vi "FormatDades.vi"(8 "Captador":refnum<vi>, 9 "Escala":u8, 10 "ValorIn":dbl, 11 "Unidades":refnum<vi>) -> (0 "NDecimals":u8, 2 "ValorOut":dbl)   [LabVIEW 2017]
panel:
  out "Value":u16
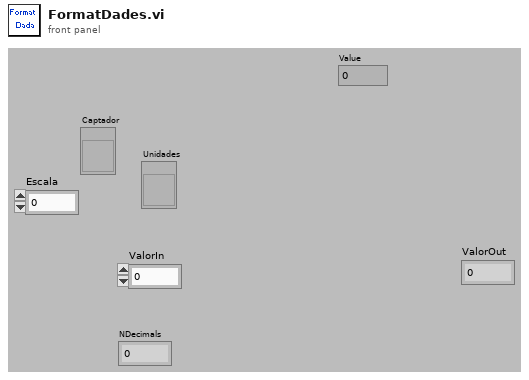
[diagram p1: front panel]
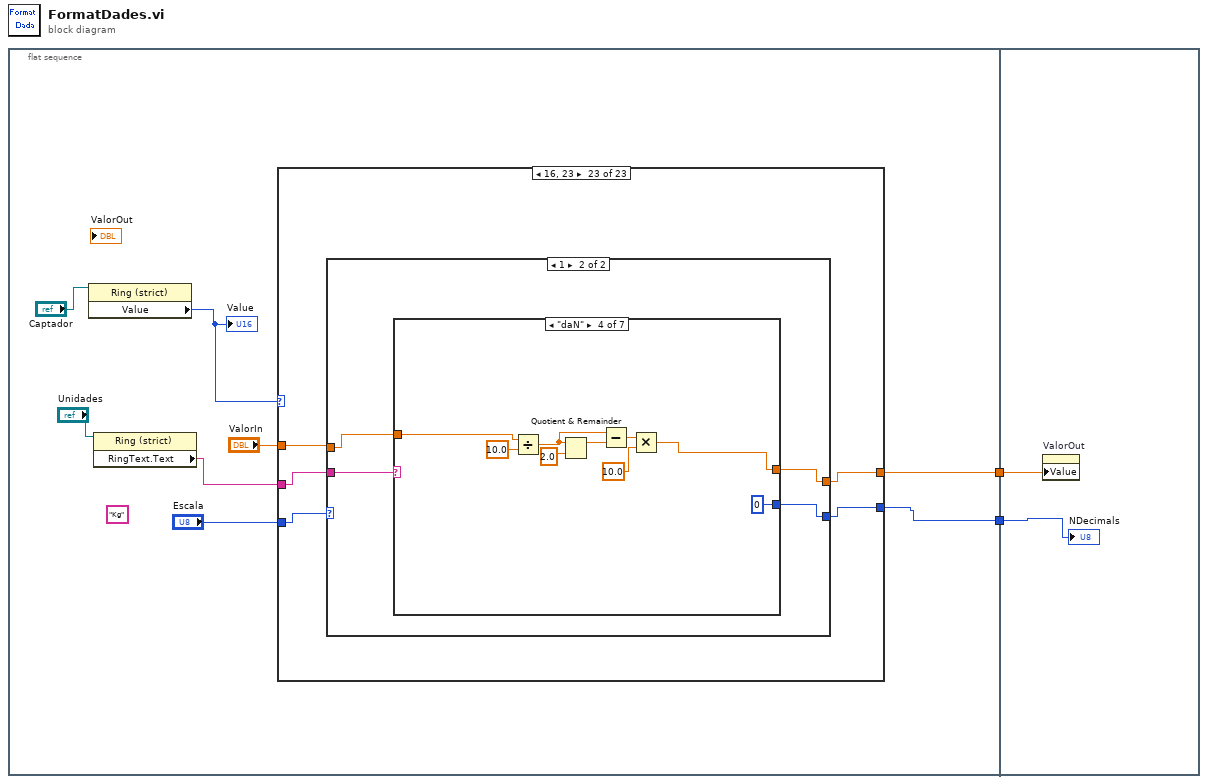
[diagram p0: block diagram]
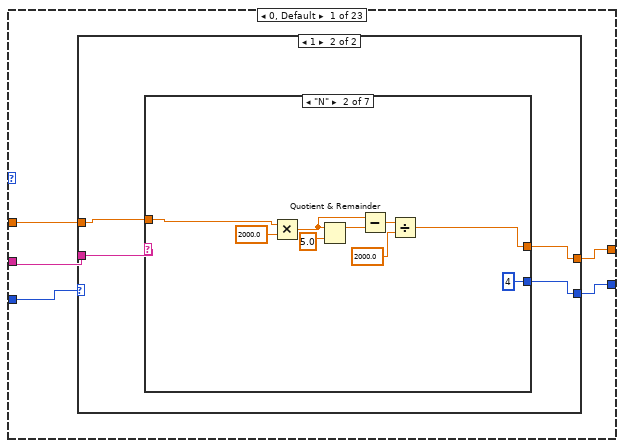
[diagram p2: hidden frame]
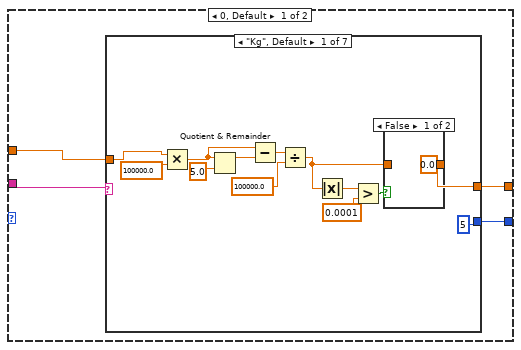
[diagram p3: hidden frame]
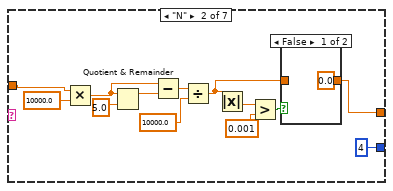
[diagram p5: hidden frame]
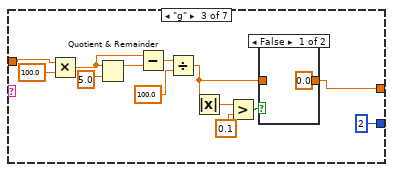
[diagram p7: hidden frame]
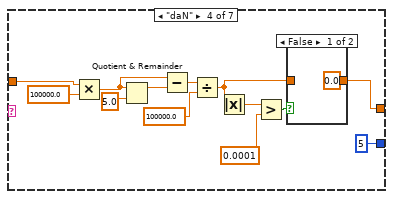
[diagram p9: hidden frame]
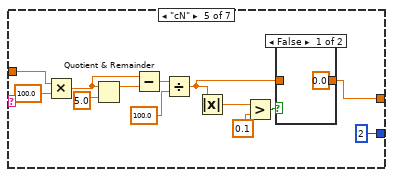
[diagram p11: hidden frame]
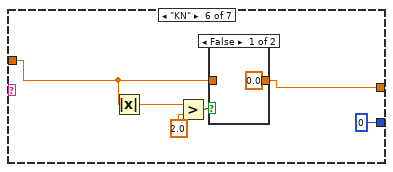
[diagram p13: hidden frame]
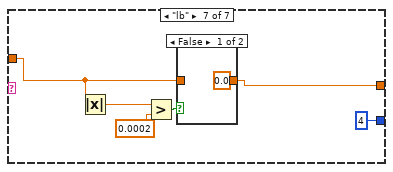
[diagram p15: hidden frame]
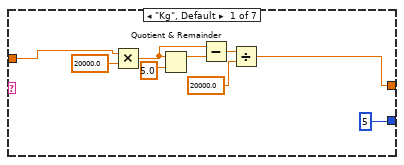
[diagram p17: hidden frame]
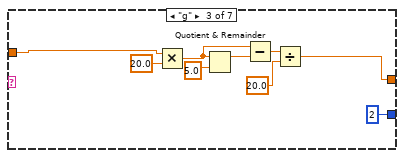
[diagram p18: hidden frame]
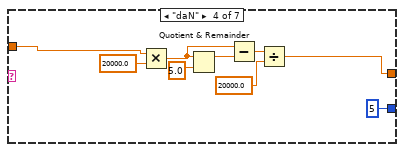
[diagram p19: hidden frame]
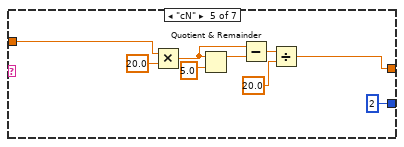
[diagram p20: hidden frame]
diagram:
  n1 = flat-sequence {
    tunnel: [w8] -> w2
    tunnel: [w3] -> w1
    tunnel: w2 -> [w3014]
    tunnel: w1 -> [w3013]
    frame #0 {
      (unwired) "Kg" ("RingText.Text")
      n2 = property class="Ring (strict)"(reference="Captador") -> ("Value"=w4:u16)  [unwired: 1 in, 2 out]
      "Value" <- w4
      n3 = property class="Ring (strict)"(reference="Unidades") -> ("RingText.Text"=w5:string)  [unwired: 1 in, 2 out]
      n4 = case shown="16, 23" w4 {
        tunnel: w5 -> [w15 w174 w293 w419 w573 w692 w819 w959 w1113 w1218 w1345 w1472 w1605 w1732 w1897 w2074 w2215 w2321 w2444 w2572 w2675 w2790 w2898]
        tunnel: [w14 w172 w291 w417 w571 w690 w816 w957 w1111 w1216 w1343 w1470 w1603 w1730 w1895 w2071 w2213 w2318 w2442 w2570 w2673 w2787 w2896] -> w8
        tunnel: "ValorIn" -> [w13 w175 w294 w420 w574 w693 w820 w960 w1114 w1219 w1346 w1473 w1606 w1733 w1898 w2075 w2216 w2322 w2445 w2573 w2676 w2791 w2899]
        tunnel: "Escala" -> [w12 w173 w292 w418 w572 w691 w818 w958 w1112 w1217 w1344 w1471 w1604 w1731 w1896 w2073 w2214 w2320 w2443 w2571 w2674 w2789 w2897]
        tunnel: [w11 w171 w290 w416 w570 w689 w817 w956 w1110 w1215 w1342 w1469 w1602 w1729 w1894 w2072 w2212 w2319 w2441 w2569 w2672 w2788 w2895] -> w3
        frame 0, Default {
          n5 = case shown="1" w12 {
            tunnel: w15 -> [w19 w113]
            tunnel: [w18 w112] -> w14
            tunnel: w13 -> [w17 w114]
            tunnel: [w16 w111] -> w11
            frame 0, Default {
              n6 = case shown="\"Kg\", Default" w19 {
                tunnel: [w21 w36 w52 w66 w81 w97 w105] -> w18
                tunnel: w17 -> [w25 w40 w55 w70 w86 w96 w104]
                tunnel: [5 4 2 5 2 0 4] -> w16
                frame "Kg", Default {
                  n7 = Multiply(x=w25, y=100000.0) -> (x*y=w28:dbl)
                  n8 = Quotient & Remainder(x=w28, y=5.0) -> (x-y*floor(x/y)=w29:dbl)  [unwired: 1 out]
                  n9 = Subtract(x=w28, y=w29) -> (x-y=w27:dbl)
                  n10 = Divide(x=w27, y=100000.0) -> (x/y=w22:dbl)
                  n11 = Absolute Value(x=w22) -> (abs(x)=w20:dbl)
                  n12 = Greater?(x=w20, y=0.0001) -> (0:w23:bool)
                  n13 = case shown="False" w23 {
                    tunnel: w22 -> [_ w34]
                    tunnel: [0.0 w34] -> w21
                    frame False {
                    }
                    frame True {
                    }
                  }
                }
                frame "N" {
                  n14 = Multiply(x=w40, y=10000.0) -> (x*y=w43:dbl)
                  n15 = Quotient & Remainder(x=w43, y=5.0) -> (x-y*floor(x/y)=w44:dbl)  [unwired: 1 out]
                  n16 = Subtract(x=w43, y=w44) -> (x-y=w42:dbl)
                  n17 = Divide(x=w42, y=10000.0) -> (x/y=w37:dbl)
                  n18 = Absolute Value(x=w37) -> (abs(x)=w35:dbl)
                  n19 = Greater?(x=w35, y=0.001) -> (0:w38:bool)
                  n20 = case shown="False" w38 {
                    tunnel: w37 -> [_ w49]
                    tunnel: [0.0 w49] -> w36
                    frame False {
                    }
                    frame True {
                    }
                  }
                }
                frame "g" {
                  n21 = Multiply(x=w55, y=100.0) -> (x*y=w58:dbl)
                  n22 = Quotient & Remainder(x=w58, y=5.0) -> (x-y*floor(x/y)=w59:dbl)  [unwired: 1 out]
                  n23 = Subtract(x=w58, y=w59) -> (x-y=w57:dbl)
                  n24 = Divide(x=w57, y=100.0) -> (x/y=w51:dbl)
                  n25 = Absolute Value(x=w51) -> (abs(x)=w50:dbl)
                  n26 = Greater?(x=w50, y=0.1) -> (0:w53:bool)
                  n27 = case shown="False" w53 {
                    tunnel: w51 -> [_ w64]
                    tunnel: [0.0 w64] -> w52
                    frame False {
                    }
                    frame True {
                    }
                  }
                }
                frame "daN" {
                  n28 = Multiply(x=w70, y=100000.0) -> (x*y=w73:dbl)
                  n29 = Quotient & Remainder(x=w73, y=5.0) -> (x-y*floor(x/y)=w74:dbl)  [unwired: 1 out]
                  n30 = Subtract(x=w73, y=w74) -> (x-y=w72:dbl)
                  n31 = Divide(x=w72, y=100000.0) -> (x/y=w67:dbl)
                  n32 = Absolute Value(x=w67) -> (abs(x)=w65:dbl)
                  n33 = Greater?(x=w65, y=0.0001) -> (0:w68:bool)
                  n34 = case shown="False" w68 {
                    tunnel: w67 -> [_ w79]
                    tunnel: [0.0 w79] -> w66
                    frame False {
                    }
                    frame True {
                    }
                  }
                }
                frame "cN" {
                  n35 = Multiply(x=w86, y=100.0) -> (x*y=w89:dbl)
                  n36 = Quotient & Remainder(x=w89, y=5.0) -> (x-y*floor(x/y)=w90:dbl)  [unwired: 1 out]
                  n37 = Subtract(x=w89, y=w90) -> (x-y=w88:dbl)
                  n38 = Divide(x=w88, y=100.0) -> (x/y=w82:dbl)
                  n39 = Absolute Value(x=w82) -> (abs(x)=w80:dbl)
                  n40 = Greater?(x=w80, y=0.1) -> (0:w83:bool)
                  n41 = case shown="False" w83 {
                    tunnel: w82 -> [_ w94]
                    tunnel: [0.0 w94] -> w81
                    frame False {
                    }
                    frame True {
                    }
                  }
                }
                frame "KN" {
                  n42 = Absolute Value(x=w96) -> (abs(x)=w95:dbl)
                  n43 = Greater?(x=w95, y=2.0) -> (0:w98:bool)
                  n44 = case shown="False" w98 {
                    tunnel: w96 -> [_ w102]
                    tunnel: [0.0 w102] -> w97
                    frame False {
                    }
                    frame True {
                    }
                  }
                }
                frame "lb" {
                  n45 = Absolute Value(x=w104) -> (abs(x)=w103:dbl)
                  n46 = Greater?(x=w103, y=0.0002) -> (0:w106:bool)
                  n47 = case shown="False" w106 {
                    tunnel: w104 -> [_ w110]
                    tunnel: [0.0 w110] -> w105
                    frame False {
                    }
                    frame True {
                    }
                  }
                }
              }
            }
            frame 1 {
              n48 = case shown="\"N\"" w113 {
                tunnel: [w115 w124 w133 w143 w153 w161 w162] -> w112
                tunnel: w114 -> [w116 w125 w134 w142 w152 w161 w163]
                tunnel: [5 4 2 5 2 0 4] -> w111
                frame "Kg", Default {
                  n49 = Multiply(x=w116, y=20000.0) -> (x*y=w119:dbl)
                  n50 = Quotient & Remainder(x=w119, y=5.0) -> (x-y*floor(x/y)=w120:dbl)  [unwired: 1 out]
                  n51 = Subtract(x=w119, y=w120) -> (x-y=w118:dbl)
                  n52 = Divide(x=w118, y=20000.0) -> (x/y=w115:dbl)
                }
                frame "N" {
                  n53 = Multiply(x=w125, y=2000.0) -> (x*y=w128:dbl)
                  n54 = Quotient & Remainder(x=w128, y=5.0) -> (x-y*floor(x/y)=w129:dbl)  [unwired: 1 out]
                  n55 = Subtract(x=w128, y=w129) -> (x-y=w127:dbl)
                  n56 = Divide(x=w127, y=2000.0) -> (x/y=w124:dbl)
                }
                frame "g" {
                  n57 = Multiply(x=w134, y=20.0) -> (x*y=w137:dbl)
                  n58 = Quotient & Remainder(x=w137, y=5.0) -> (x-y*floor(x/y)=w138:dbl)  [unwired: 1 out]
                  n59 = Subtract(x=w137, y=w138) -> (x-y=w136:dbl)
                  n60 = Divide(x=w136, y=20.0) -> (x/y=w133:dbl)
                }
                frame "daN" {
                  n61 = Multiply(x=w142, y=20000.0) -> (x*y=w146:dbl)
                  n62 = Quotient & Remainder(x=w146, y=5.0) -> (x-y*floor(x/y)=w147:dbl)  [unwired: 1 out]
                  n63 = Subtract(x=w146, y=w147) -> (x-y=w145:dbl)
                  n64 = Divide(x=w145, y=20000.0) -> (x/y=w143:dbl)
                }
                frame "cN" {
                  n65 = Multiply(x=w152, y=20.0) -> (x*y=w156:dbl)
                  n66 = Quotient & Remainder(x=w156, y=5.0) -> (x-y*floor(x/y)=w157:dbl)  [unwired: 1 out]
                  n67 = Subtract(x=w156, y=w157) -> (x-y=w155:dbl)
                  n68 = Divide(x=w155, y=20.0) -> (x/y=w153:dbl)
                }
                frame "KN" {
                }
                frame "lb" {
                  n69 = Multiply(x=w163, y=10000.0) -> (x*y=w166:dbl)
                  n70 = Quotient & Remainder(x=w166, y=5.0) -> (x-y*floor(x/y)=w167:dbl)  [unwired: 1 out]
                  n71 = Subtract(x=w166, y=w167) -> (x-y=w165:dbl)
                  n72 = Divide(x=w165, y=10000.0) -> (x/y=w162:dbl)
                }
              }
            }
          }
        }
        frame 1 {
          n73 = case shown="0, Default" w173 {
            tunnel: [w179 w240] -> w172
            tunnel: [w178 w239] -> w171
            tunnel: w175 -> [w177 w238]
            tunnel: w174 -> [w176 w237]
            frame 0, Default {
              n74 = case shown="\"Kg\", Default" w176 {
                tunnel: [w181 w189 w197 w205 w213 w220 w223] -> w179
                tunnel: [4 3 1 4 1 0 4] -> w178
                tunnel: w177 -> [w182 w190 w198 w206 w214 w220 w227]
                frame "Kg", Default {
                  n75 = Absolute Value(x=w182) -> (abs(x)=w180:dbl)
                  n76 = Greater?(x=w180, y=0.0002) -> (0:w183:bool)
                  n77 = case shown="False" w183 {
                    tunnel: w182 -> [_ w187]
                    tunnel: [0.0 w187] -> w181
                    frame False {
                    }
                    frame True {
                    }
                  }
                }
                frame "N" {
                  n78 = Absolute Value(x=w190) -> (abs(x)=w188:dbl)
                  n79 = Greater?(x=w188, y=0.002) -> (0:w191:bool)
                  n80 = case shown="False" w191 {
                    tunnel: w190 -> [_ w195]
                    tunnel: [0.0 w195] -> w189
                    frame False {
                    }
                    frame True {
                    }
                  }
                }
                frame "g" {
                  n81 = Absolute Value(x=w198) -> (abs(x)=w196:dbl)
                  n82 = Greater?(x=w196, y=2.0) -> (0:w199:bool)
                  n83 = case shown="False" w199 {
                    tunnel: w198 -> [_ w203]
                    tunnel: [0.0 w203] -> w197
                    frame False {
                    }
                    frame True {
                    }
                  }
                }
                frame "daN" {
                  n84 = Absolute Value(x=w206) -> (abs(x)=w204:dbl)
                  n85 = Greater?(x=w204, y=0.0002) -> (0:w207:bool)
                  n86 = case shown="False" w207 {
                    tunnel: w206 -> [_ w211]
                    tunnel: [0.0 w211] -> w205
                    frame False {
                    }
                    frame True {
                    }
                  }
                }
                frame "cN" {
                  n87 = Absolute Value(x=w214) -> (abs(x)=w212:dbl)
                  n88 = Greater?(x=w212, y=2.0) -> (0:w215:bool)
                  n89 = case shown="False" w215 {
                    tunnel: w214 -> [_ w219]
                    tunnel: [0.0 w219] -> w213
                    frame False {
                    }
                    frame True {
                    }
                  }
                }
                frame "KN" {
                }
                frame "lb" {
                  n90 = Multiply(x=w227, y=10000.0) -> (x*y=w230:dbl)
                  n91 = Quotient & Remainder(x=w230, y=2.0) -> (x-y*floor(x/y)=w231:dbl)  [unwired: 1 out]
                  n92 = Subtract(x=w230, y=w231) -> (x-y=w229:dbl)
                  n93 = Divide(x=w229, y=10000.0) -> (x/y=w224:dbl)
                  n94 = Absolute Value(x=w224) -> (abs(x)=w222:dbl)
                  n95 = Greater?(x=w222, y=0.0004) -> (0:w225:bool)
                  n96 = case shown="False" w225 {
                    tunnel: w224 -> [_ w236]
                    tunnel: [0.0 w236] -> w223
                    frame False {
                    }
                    frame True {
                    }
                  }
                }
              }
            }
            frame 1 {
              n97 = case shown="\"N\"" w237 {
                tunnel: [w242 w250 w260 w268 w278 w286 w288] -> w240
                tunnel: [4 3 1 4 1 0 3] -> w239
                tunnel: w238 -> [w241 w251 w259 w269 w277 w286 w288]
                frame "Kg", Default {
                  n98 = Multiply(x=w241, y=10000.0) -> (x*y=w245:dbl)
                  n99 = Quotient & Remainder(x=w245, y=5.0) -> (x-y*floor(x/y)=w246:dbl)  [unwired: 1 out]
                  n100 = Subtract(x=w245, y=w246) -> (x-y=w244:dbl)
                  n101 = Divide(x=w244, y=10000.0) -> (x/y=w242:dbl)
                }
                frame "N" {
                  n102 = Multiply(x=w251, y=1000.0) -> (x*y=w254:dbl)
                  n103 = Quotient & Remainder(x=w254, y=5.0) -> (x-y*floor(x/y)=w255:dbl)  [unwired: 1 out]
                  n104 = Subtract(x=w254, y=w255) -> (x-y=w253:dbl)
                  n105 = Divide(x=w253, y=1000.0) -> (x/y=w250:dbl)
                }
                frame "g" {
                  n106 = Multiply(x=w259, y=10.0) -> (x*y=w263:dbl)
                  n107 = Quotient & Remainder(x=w263, y=5.0) -> (x-y*floor(x/y)=w264:dbl)  [unwired: 1 out]
                  n108 = Subtract(x=w263, y=w264) -> (x-y=w262:dbl)
                  n109 = Divide(x=w262, y=10.0) -> (x/y=w260:dbl)
                }
                frame "daN" {
                  n110 = Multiply(x=w269, y=10000.0) -> (x*y=w272:dbl)
                  n111 = Quotient & Remainder(x=w272, y=5.0) -> (x-y*floor(x/y)=w273:dbl)  [unwired: 1 out]
                  n112 = Subtract(x=w272, y=w273) -> (x-y=w271:dbl)
                  n113 = Divide(x=w271, y=10000.0) -> (x/y=w268:dbl)
                }
                frame "cN" {
                  n114 = Multiply(x=w277, y=10.0) -> (x*y=w281:dbl)
                  n115 = Quotient & Remainder(x=w281, y=5.0) -> (x-y*floor(x/y)=w282:dbl)  [unwired: 1 out]
                  n116 = Subtract(x=w281, y=w282) -> (x-y=w280:dbl)
                  n117 = Divide(x=w280, y=10.0) -> (x/y=w278:dbl)
                }
                frame "KN" {
                }
                frame "lb" {
                }
              }
            }
          }
        }
        frame 2 {
          n118 = case shown="0, Default" w292 {
            tunnel: [w298 w394] -> w291
            tunnel: [w297 w393] -> w290
            tunnel: w294 -> [w296 w392]
            tunnel: w293 -> [w295 w391]
            frame 0, Default {
              n119 = case shown="\"lb\"" w295 {
                tunnel: [w300 w315 w330 w345 w361 w374 w377] -> w298
                tunnel: [4 3 1 4 1 0 4] -> w297
                tunnel: w296 -> [w304 w319 w334 w349 w364 w374 w381]
                frame "Kg", Default {
                  n120 = Multiply(x=w304, y=10000.0) -> (x*y=w307:dbl)
                  n121 = Quotient & Remainder(x=w307, y=2.0) -> (x-y*floor(x/y)=w308:dbl)  [unwired: 1 out]
                  n122 = Subtract(x=w307, y=w308) -> (x-y=w306:dbl)
                  n123 = Divide(x=w306, y=10000.0) -> (x/y=w301:dbl)
                  n124 = Absolute Value(x=w301) -> (abs(x)=w299:dbl)
                  n125 = Greater?(x=w299, y=0.0004) -> (0:w302:bool)
                  n126 = case shown="False" w302 {
                    tunnel: w301 -> [_ w313]
                    tunnel: [0.0 w313] -> w300
                    frame False {
                    }
                    frame True {
                    }
                  }
                }
                frame "N" {
                  n127 = Multiply(x=w319, y=1000.0) -> (x*y=w322:dbl)
                  n128 = Quotient & Remainder(x=w322, y=2.0) -> (x-y*floor(x/y)=w323:dbl)  [unwired: 1 out]
                  n129 = Subtract(x=w322, y=w323) -> (x-y=w321:dbl)
                  n130 = Divide(x=w321, y=1000.0) -> (x/y=w316:dbl)
                  n131 = Absolute Value(x=w316) -> (abs(x)=w314:dbl)
                  n132 = Greater?(x=w314, y=0.004) -> (0:w317:bool)
                  n133 = case shown="False" w317 {
                    tunnel: w316 -> [_ w328]
                    tunnel: [0.0 w328] -> w315
                    frame False {
                    }
                    frame True {
                    }
                  }
                }
                frame "g" {
                  n134 = Multiply(x=w334, y=10.0) -> (x*y=w337:dbl)
                  n135 = Quotient & Remainder(x=w337, y=2.0) -> (x-y*floor(x/y)=w338:dbl)  [unwired: 1 out]
                  n136 = Subtract(x=w337, y=w338) -> (x-y=w336:dbl)
                  n137 = Divide(x=w336, y=10.0) -> (x/y=w331:dbl)
                  n138 = Absolute Value(x=w331) -> (abs(x)=w329:dbl)
                  n139 = Greater?(x=w329, y=0.4) -> (0:w332:bool)
                  n140 = case shown="False" w332 {
                    tunnel: w331 -> [_ w343]
                    tunnel: [0.0 w343] -> w330
                    frame False {
                    }
                    frame True {
                    }
                  }
                }
                frame "daN" {
                  n141 = Multiply(x=w349, y=10000.0) -> (x*y=w352:dbl)
                  n142 = Quotient & Remainder(x=w352, y=2.0) -> (x-y*floor(x/y)=w353:dbl)  [unwired: 1 out]
                  n143 = Subtract(x=w352, y=w353) -> (x-y=w351:dbl)
                  n144 = Divide(x=w351, y=10000.0) -> (x/y=w346:dbl)
                  n145 = Absolute Value(x=w346) -> (abs(x)=w344:dbl)
                  n146 = Greater?(x=w344, y=0.0004) -> (0:w347:bool)
                  n147 = case shown="False" w347 {
                    tunnel: w346 -> [_ w358]
                    tunnel: [0.0 w358] -> w345
                    frame False {
                    }
                    frame True {
                    }
                  }
                }
                frame "cN" {
                  n148 = Multiply(x=w364, y=10.0) -> (x*y=w367:dbl)
                  n149 = Quotient & Remainder(x=w367, y=2.0) -> (x-y*floor(x/y)=w368:dbl)  [unwired: 1 out]
                  n150 = Subtract(x=w367, y=w368) -> (x-y=w366:dbl)
                  n151 = Divide(x=w366, y=10.0) -> (x/y=w360:dbl)
                  n152 = Absolute Value(x=w360) -> (abs(x)=w359:dbl)
                  n153 = Greater?(x=w359, y=0.4) -> (0:w362:bool)
                  n154 = case shown="False" w362 {
                    tunnel: w360 -> [_ w373]
                    tunnel: [0.0 w373] -> w361
                    frame False {
                    }
                    frame True {
                    }
                  }
                }
                frame "KN" {
                }
                frame "lb" {
                  n155 = Multiply(x=w381, y=10000.0) -> (x*y=w384:dbl)
                  n156 = Quotient & Remainder(x=w384, y=5.0) -> (x-y*floor(x/y)=w385:dbl)  [unwired: 1 out]
                  n157 = Subtract(x=w384, y=w385) -> (x-y=w383:dbl)
                  n158 = Divide(x=w383, y=10000.0) -> (x/y=w378:dbl)
                  n159 = Absolute Value(x=w378) -> (abs(x)=w376:dbl)
                  n160 = Greater?(x=w376, y=0.001) -> (0:w379:bool)
                  n161 = case shown="False" w379 {
                    tunnel: w378 -> [_ w390]
                    tunnel: [0.0 w390] -> w377
                    frame False {
                    }
                    frame True {
                    }
                  }
                }
              }
            }
            frame 1 {
              n162 = case shown="\"Kg\", Default" w391 {
                tunnel: [w395 w397 w399 w401 w403 w405 w408] -> w394
                tunnel: [3 2 0 3 0 0 4] -> w393
                tunnel: w392 -> [w395 w397 w399 w401 w403 w405 w407]
                frame "Kg", Default {
                }
                frame "N" {
                }
                frame "g" {
                }
                frame "daN" {
                }
                frame "cN" {
                }
                frame "KN" {
                }
                frame "lb" {
                  n163 = Multiply(x=w407, y=2000.0) -> (x*y=w411:dbl)
                  n164 = Quotient & Remainder(x=w411, y=5.0) -> (x-y*floor(x/y)=w412:dbl)  [unwired: 1 out]
                  n165 = Subtract(x=w411, y=w412) -> (x-y=w410:dbl)
                  n166 = Divide(x=w410, y=2000.0) -> (x/y=w408:dbl)
                }
              }
            }
          }
        }
        frame 3 {
          n167 = case shown="0, Default" w418 {
            tunnel: w419 -> [w424 w513]
            tunnel: [w423 w512] -> w417
            tunnel: [w422 w511] -> w416
            tunnel: w420 -> [w421 w510]
            frame 0, Default {
              n168 = case shown="\"Kg\", Default" w424 {
                tunnel: [w426 w441 w456 w471 w486 w500 w503] -> w423
                tunnel: [4 3 1 4 1 0 3] -> w422
                tunnel: w421 -> [w430 w445 w460 w475 w490 w500 w504]
                frame "Kg", Default {
                  n169 = Multiply(x=w430, y=10000.0) -> (x*y=w433:dbl)
                  n170 = Quotient & Remainder(x=w433, y=5.0) -> (x-y*floor(x/y)=w434:dbl)  [unwired: 1 out]
                  n171 = Subtract(x=w433, y=w434) -> (x-y=w432:dbl)
                  n172 = Divide(x=w432, y=10000.0) -> (x/y=w427:dbl)
                  n173 = Absolute Value(x=w427) -> (abs(x)=w425:dbl)
                  n174 = Greater?(x=w425, y=0.001) -> (0:w428:bool)
                  n175 = case shown="False" w428 {
                    tunnel: w427 -> [_ w439]
                    tunnel: [0.0 w439] -> w426
                    frame False {
                    }
                    frame True {
                    }
                  }
                }
                frame "N" {
                  n176 = Multiply(x=w445, y=1000.0) -> (x*y=w448:dbl)
                  n177 = Quotient & Remainder(x=w448, y=5.0) -> (x-y*floor(x/y)=w449:dbl)  [unwired: 1 out]
                  n178 = Subtract(x=w448, y=w449) -> (x-y=w447:dbl)
                  n179 = Divide(x=w447, y=1000.0) -> (x/y=w442:dbl)
                  n180 = Absolute Value(x=w442) -> (abs(x)=w440:dbl)
                  n181 = Greater?(x=w440, y=0.01) -> (0:w443:bool)
                  n182 = case shown="False" w443 {
                    tunnel: w442 -> [_ w454]
                    tunnel: [0.0 w454] -> w441
                    frame False {
                    }
                    frame True {
                    }
                  }
                }
                frame "g" {
                  n183 = Multiply(x=w460, y=10.0) -> (x*y=w463:dbl)
                  n184 = Quotient & Remainder(x=w463, y=5.0) -> (x-y*floor(x/y)=w464:dbl)  [unwired: 1 out]
                  n185 = Subtract(x=w463, y=w464) -> (x-y=w462:dbl)
                  n186 = Divide(x=w462, y=10.0) -> (x/y=w457:dbl)
                  n187 = Absolute Value(x=w457) -> (abs(x)=w455:dbl)
                  n188 = Greater?(x=w455, y=1.0) -> (0:w458:bool)
                  n189 = case shown="False" w458 {
                    tunnel: w457 -> [_ w469]
                    tunnel: [0.0 w469] -> w456
                    frame False {
                    }
                    frame True {
                    }
                  }
                }
                frame "daN" {
                  n190 = Multiply(x=w475, y=10000.0) -> (x*y=w478:dbl)
                  n191 = Quotient & Remainder(x=w478, y=5.0) -> (x-y*floor(x/y)=w479:dbl)  [unwired: 1 out]
                  n192 = Subtract(x=w478, y=w479) -> (x-y=w477:dbl)
                  n193 = Divide(x=w477, y=10000.0) -> (x/y=w472:dbl)
                  n194 = Absolute Value(x=w472) -> (abs(x)=w470:dbl)
                  n195 = Greater?(x=w470, y=0.001) -> (0:w473:bool)
                  n196 = case shown="False" w473 {
                    tunnel: w472 -> [_ w484]
                    tunnel: [0.0 w484] -> w471
                    frame False {
                    }
                    frame True {
                    }
                  }
                }
                frame "cN" {
                  n197 = Multiply(x=w490, y=10.0) -> (x*y=w494:dbl)
                  n198 = Quotient & Remainder(x=w494, y=5.0) -> (x-y*floor(x/y)=w495:dbl)  [unwired: 1 out]
                  n199 = Subtract(x=w494, y=w495) -> (x-y=w493:dbl)
                  n200 = Divide(x=w493, y=10.0) -> (x/y=w487:dbl)
                  n201 = Absolute Value(x=w487) -> (abs(x)=w485:dbl)
                  n202 = Greater?(x=w485, y=1.0) -> (0:w488:bool)
                  n203 = case shown="False" w488 {
                    tunnel: w487 -> [_ w499]
                    tunnel: [0.0 w499] -> w486
                    frame False {
                    }
                    frame True {
                    }
                  }
                }
                frame "KN" {
                }
                frame "lb" {
                  n204 = Absolute Value(x=w504) -> (abs(x)=w502:dbl)
                  n205 = Greater?(x=w502, y=0.002) -> (0:w505:bool)
                  n206 = case shown="False" w505 {
                    tunnel: w504 -> [_ w509]
                    tunnel: [0.0 w509] -> w503
                    frame False {
                    }
                    frame True {
                    }
                  }
                }
              }
            }
            frame 1 {
              n207 = case shown="\"lb\"" w513 {
                tunnel: [w515 w524 w533 w542 w552 w559 w562] -> w512
                tunnel: [4 3 1 4 2 0 3] -> w511
                tunnel: w510 -> [w514 w523 w532 w541 w550 w559 w561]
                frame "Kg", Default {
                  n208 = Multiply(x=w514, y=2000.0) -> (x*y=w518:dbl)
                  n209 = Quotient & Remainder(x=w518, y=5.0) -> (x-y*floor(x/y)=w519:dbl)  [unwired: 1 out]
                  n210 = Subtract(x=w518, y=w519) -> (x-y=w517:dbl)
                  n211 = Divide(x=w517, y=2000.0) -> (x/y=w515:dbl)
                }
                frame "N" {
                  n212 = Multiply(x=w523, y=200.0) -> (x*y=w527:dbl)
                  n213 = Quotient & Remainder(x=w527, y=5.0) -> (x-y*floor(x/y)=w528:dbl)  [unwired: 1 out]
                  n214 = Subtract(x=w527, y=w528) -> (x-y=w526:dbl)
                  n215 = Divide(x=w526, y=200.0) -> (x/y=w524:dbl)
                }
                frame "g" {
                  n216 = Multiply(x=w532, y=2.0) -> (x*y=w536:dbl)
                  n217 = Quotient & Remainder(x=w536, y=5.0) -> (x-y*floor(x/y)=w537:dbl)  [unwired: 1 out]
                  n218 = Subtract(x=w536, y=w537) -> (x-y=w535:dbl)
                  n219 = Divide(x=w535, y=2.0) -> (x/y=w533:dbl)
                }
                frame "daN" {
                  n220 = Multiply(x=w541, y=2000.0) -> (x*y=w545:dbl)
                  n221 = Quotient & Remainder(x=w545, y=5.0) -> (x-y*floor(x/y)=w546:dbl)  [unwired: 1 out]
                  n222 = Subtract(x=w545, y=w546) -> (x-y=w544:dbl)
                  n223 = Divide(x=w544, y=2000.0) -> (x/y=w542:dbl)
                }
                frame "cN" {
                  n224 = Multiply(x=w550, y=2.0) -> (x*y=w555:dbl)
                  n225 = Quotient & Remainder(x=w555, y=5.0) -> (x-y*floor(x/y)=w556:dbl)  [unwired: 1 out]
                  n226 = Subtract(x=w555, y=w556) -> (x-y=w554:dbl)
                  n227 = Divide(x=w554, y=2.0) -> (x/y=w552:dbl)
                }
                frame "KN" {
                }
                frame "lb" {
                  n228 = Multiply(x=w561, y=1000.0) -> (x*y=w565:dbl)
                  n229 = Quotient & Remainder(x=w565, y=5.0) -> (x-y*floor(x/y)=w566:dbl)  [unwired: 1 out]
                  n230 = Subtract(x=w565, y=w566) -> (x-y=w564:dbl)
                  n231 = Divide(x=w564, y=1000.0) -> (x/y=w562:dbl)
                }
              }
            }
          }
        }
        frame 4 {
          n232 = case shown="0, Default" w572 {
            tunnel: [w578 w639] -> w571
            tunnel: [w577 w638] -> w570
            tunnel: w574 -> [w576 w637]
            tunnel: w573 -> [w575 w636]
            frame 0, Default {
              n233 = case shown="\"Kg\", Default" w575 {
                tunnel: [w580 w588 w596 w604 w612 w619 w622] -> w578
                tunnel: [3 2 0 3 0 0 3] -> w577
                tunnel: w576 -> [w581 w589 w597 w605 w613 w619 w626]
                frame "Kg", Default {
                  n234 = Absolute Value(x=w581) -> (abs(x)=w579:dbl)
                  n235 = Greater?(x=w579, y=0.002) -> (0:w582:bool)
                  n236 = case shown="False" w582 {
                    tunnel: w581 -> [_ w586]
                    tunnel: [0.0 w586] -> w580
                    frame False {
                    }
                    frame True {
                    }
                  }
                }
                frame "N" {
                  n237 = Absolute Value(x=w589) -> (abs(x)=w587:dbl)
                  n238 = Greater?(x=w587, y=0.02) -> (0:w590:bool)
                  n239 = case shown="False" w590 {
                    tunnel: w589 -> [_ w594]
                    tunnel: [0.0 w594] -> w588
                    frame False {
                    }
                    frame True {
                    }
                  }
                }
                frame "g" {
                  n240 = Absolute Value(x=w597) -> (abs(x)=w595:dbl)
                  n241 = Greater?(x=w595, y=2.0) -> (0:w598:bool)
                  n242 = case shown="False" w598 {
                    tunnel: w597 -> [_ w602]
                    tunnel: [0.0 w602] -> w596
                    frame False {
                    }
                    frame True {
                    }
                  }
                }
                frame "daN" {
                  n243 = Absolute Value(x=w605) -> (abs(x)=w603:dbl)
                  n244 = Greater?(x=w603, y=0.002) -> (0:w606:bool)
                  n245 = case shown="False" w606 {
                    tunnel: w605 -> [_ w610]
                    tunnel: [0.0 w610] -> w604
                    frame False {
                    }
                    frame True {
                    }
                  }
                }
                frame "cN" {
                  n246 = Absolute Value(x=w613) -> (abs(x)=w611:dbl)
                  n247 = Greater?(x=w611, y=2.0) -> (0:w614:bool)
                  n248 = case shown="False" w614 {
                    tunnel: w613 -> [_ w618]
                    tunnel: [0.0 w618] -> w612
                    frame False {
                    }
                    frame True {
                    }
                  }
                }
                frame "KN" {
                }
                frame "lb" {
                  n249 = Multiply(x=w626, y=1000.0) -> (x*y=w629:dbl)
                  n250 = Quotient & Remainder(x=w629, y=2.0) -> (x-y*floor(x/y)=w630:dbl)  [unwired: 1 out]
                  n251 = Subtract(x=w629, y=w630) -> (x-y=w628:dbl)
                  n252 = Divide(x=w628, y=1000.0) -> (x/y=w623:dbl)
                  n253 = Absolute Value(x=w623) -> (abs(x)=w621:dbl)
                  n254 = Greater?(x=w621, y=0.004) -> (0:w624:bool)
                  n255 = case shown="False" w624 {
                    tunnel: w623 -> [_ w635]
                    tunnel: [0.0 w635] -> w622
                    frame False {
                    }
                    frame True {
                    }
                  }
                }
              }
            }
            frame 1 {
              n256 = case shown="\"lb\"" w636 {
                tunnel: [w641 w649 w659 w667 w677 w685 w687] -> w639
                tunnel: [3 2 0 3 0 0 2] -> w638
                tunnel: w637 -> [w640 w650 w658 w668 w676 w685 w687]
                frame "Kg", Default {
                  n257 = Multiply(x=w640, y=1000.0) -> (x*y=w644:dbl)
                  n258 = Quotient & Remainder(x=w644, y=5.0) -> (x-y*floor(x/y)=w645:dbl)  [unwired: 1 out]
                  n259 = Subtract(x=w644, y=w645) -> (x-y=w643:dbl)
                  n260 = Divide(x=w643, y=1000.0) -> (x/y=w641:dbl)
                }
                frame "N" {
                  n261 = Multiply(x=w650, y=100.0) -> (x*y=w653:dbl)
                  n262 = Quotient & Remainder(x=w653, y=5.0) -> (x-y*floor(x/y)=w654:dbl)  [unwired: 1 out]
                  n263 = Subtract(x=w653, y=w654) -> (x-y=w652:dbl)
                  n264 = Divide(x=w652, y=100.0) -> (x/y=w649:dbl)
                }
                frame "g" {
                  n265 = Multiply(x=w658, y=1.0) -> (x*y=w662:dbl)
                  n266 = Quotient & Remainder(x=w662, y=5.0) -> (x-y*floor(x/y)=w663:dbl)  [unwired: 1 out]
                  n267 = Subtract(x=w662, y=w663) -> (x-y=w661:dbl)
                  n268 = Divide(x=w661, y=1.0) -> (x/y=w659:dbl)
                }
                frame "daN" {
                  n269 = Multiply(x=w668, y=1000.0) -> (x*y=w671:dbl)
                  n270 = Quotient & Remainder(x=w671, y=5.0) -> (x-y*floor(x/y)=w672:dbl)  [unwired: 1 out]
                  n271 = Subtract(x=w671, y=w672) -> (x-y=w670:dbl)
                  n272 = Divide(x=w670, y=1000.0) -> (x/y=w667:dbl)
                }
                frame "cN" {
                  n273 = Multiply(x=w676, y=1.0) -> (x*y=w680:dbl)
                  n274 = Quotient & Remainder(x=w680, y=5.0) -> (x-y*floor(x/y)=w681:dbl)  [unwired: 1 out]
                  n275 = Subtract(x=w680, y=w681) -> (x-y=w679:dbl)
                  n276 = Divide(x=w679, y=1.0) -> (x/y=w677:dbl)
                }
                frame "KN" {
                }
                frame "lb" {
                }
              }
            }
          }
        }
        frame 17 {
          n277 = case shown="0, Default" w691 {
            tunnel: [w697 w758] -> w690
            tunnel: [w696 w757] -> w689
            tunnel: w693 -> [w695 w756]
            tunnel: w692 -> [w694 w755]
            frame 0, Default {
              n278 = case shown="\"Kg\", Default" w694 {
                tunnel: [w699 w707 w715 w723 w731 w738 w741] -> w697
                tunnel: [3 2 0 3 0 0 3] -> w696
                tunnel: w695 -> [w700 w708 w716 w724 w732 w738 w745]
                frame "Kg", Default {
                  n279 = Absolute Value(x=w700) -> (abs(x)=w698:dbl)
                  n280 = Greater?(x=w698, y=0.002) -> (0:w701:bool)
                  n281 = case shown="False" w701 {
                    tunnel: w700 -> [_ w705]
                    tunnel: [0.0 w705] -> w699
                    frame False {
                    }
                    frame True {
                    }
                  }
                }
                frame "N" {
                  n282 = Absolute Value(x=w708) -> (abs(x)=w706:dbl)
                  n283 = Greater?(x=w706, y=0.02) -> (0:w709:bool)
                  n284 = case shown="False" w709 {
                    tunnel: w708 -> [_ w713]
                    tunnel: [0.0 w713] -> w707
                    frame False {
                    }
                    frame True {
                    }
                  }
                }
                frame "g" {
                  n285 = Absolute Value(x=w716) -> (abs(x)=w714:dbl)
                  n286 = Greater?(x=w714, y=2.0) -> (0:w717:bool)
                  n287 = case shown="False" w717 {
                    tunnel: w716 -> [_ w721]
                    tunnel: [0.0 w721] -> w715
                    frame False {
                    }
                    frame True {
                    }
                  }
                }
                frame "daN" {
                  n288 = Absolute Value(x=w724) -> (abs(x)=w722:dbl)
                  n289 = Greater?(x=w722, y=0.002) -> (0:w725:bool)
                  n290 = case shown="False" w725 {
                    tunnel: w724 -> [_ w729]
                    tunnel: [0.0 w729] -> w723
                    frame False {
                    }
                    frame True {
                    }
                  }
                }
                frame "cN" {
                  n291 = Absolute Value(x=w732) -> (abs(x)=w730:dbl)
                  n292 = Greater?(x=w730, y=2.0) -> (0:w733:bool)
                  n293 = case shown="False" w733 {
                    tunnel: w732 -> [_ w737]
                    tunnel: [0.0 w737] -> w731
                    frame False {
                    }
                    frame True {
                    }
                  }
                }
                frame "KN" {
                }
                frame "lb" {
                  n294 = Multiply(x=w745, y=1000.0) -> (x*y=w748:dbl)
                  n295 = Quotient & Remainder(x=w748, y=2.0) -> (x-y*floor(x/y)=w749:dbl)  [unwired: 1 out]
                  n296 = Subtract(x=w748, y=w749) -> (x-y=w747:dbl)
                  n297 = Divide(x=w747, y=1000.0) -> (x/y=w742:dbl)
                  n298 = Absolute Value(x=w742) -> (abs(x)=w740:dbl)
                  n299 = Greater?(x=w740, y=0.004) -> (0:w743:bool)
                  n300 = case shown="False" w743 {
                    tunnel: w742 -> [_ w754]
                    tunnel: [0.0 w754] -> w741
                    frame False {
                    }
                    frame True {
                    }
                  }
                }
              }
            }
            frame 1 {
              n301 = case shown="\"Kg\", Default" w755 {
                tunnel: [w760 w768 w776 w784 w792 w799 w802] -> w758
                tunnel: [3 2 0 3 0 0 3] -> w757
                tunnel: w756 -> [w761 w769 w777 w785 w793 w799 w806]
                frame "Kg", Default {
                  n302 = Absolute Value(x=w761) -> (abs(x)=w759:dbl)
                  n303 = Greater?(x=w759, y=0.002) -> (0:w762:bool)
                  n304 = case shown="False" w762 {
                    tunnel: w761 -> [_ w766]
                    tunnel: [0.0 w766] -> w760
                    frame False {
                    }
                    frame True {
                    }
                  }
                }
                frame "N" {
                  n305 = Absolute Value(x=w769) -> (abs(x)=w767:dbl)
                  n306 = Greater?(x=w767, y=0.02) -> (0:w770:bool)
                  n307 = case shown="False" w770 {
                    tunnel: w769 -> [_ w774]
                    tunnel: [0.0 w774] -> w768
                    frame False {
                    }
                    frame True {
                    }
                  }
                }
                frame "g" {
                  n308 = Absolute Value(x=w777) -> (abs(x)=w775:dbl)
                  n309 = Greater?(x=w775, y=2.0) -> (0:w778:bool)
                  n310 = case shown="False" w778 {
                    tunnel: w777 -> [_ w782]
                    tunnel: [0.0 w782] -> w776
                    frame False {
                    }
                    frame True {
                    }
                  }
                }
                frame "daN" {
                  n311 = Absolute Value(x=w785) -> (abs(x)=w783:dbl)
                  n312 = Greater?(x=w783, y=0.002) -> (0:w786:bool)
                  n313 = case shown="False" w786 {
                    tunnel: w785 -> [_ w790]
                    tunnel: [0.0 w790] -> w784
                    frame False {
                    }
                    frame True {
                    }
                  }
                }
                frame "cN" {
                  n314 = Absolute Value(x=w793) -> (abs(x)=w791:dbl)
                  n315 = Greater?(x=w791, y=2.0) -> (0:w794:bool)
                  n316 = case shown="False" w794 {
                    tunnel: w793 -> [_ w798]
                    tunnel: [0.0 w798] -> w792
                    frame False {
                    }
                    frame True {
                    }
                  }
                }
                frame "KN" {
                }
                frame "lb" {
                  n317 = Multiply(x=w806, y=1000.0) -> (x*y=w809:dbl)
                  n318 = Quotient & Remainder(x=w809, y=2.0) -> (x-y*floor(x/y)=w810:dbl)  [unwired: 1 out]
                  n319 = Subtract(x=w809, y=w810) -> (x-y=w808:dbl)
                  n320 = Divide(x=w808, y=1000.0) -> (x/y=w803:dbl)
                  n321 = Absolute Value(x=w803) -> (abs(x)=w801:dbl)
                  n322 = Greater?(x=w801, y=0.004) -> (0:w804:bool)
                  n323 = case shown="False" w804 {
                    tunnel: w803 -> [_ w815]
                    tunnel: [0.0 w815] -> w802
                    frame False {
                    }
                    frame True {
                    }
                  }
                }
              }
            }
          }
        }
        frame 5 {
          n324 = case shown="0, Default" w818 {
            tunnel: [w824 w920] -> w816
            tunnel: [w823 w919] -> w817
            tunnel: w820 -> [w822 w918]
            tunnel: w819 -> [w821 w917]
            frame 0, Default {
              n325 = case shown="\"Kg\", Default" w821 {
                tunnel: [w826 w842 w857 w872 w887 w900 w904] -> w824
                tunnel: [3 2 0 3 0 0 3] -> w823
                tunnel: w822 -> [w830 w845 w860 w875 w890 w900 w907]
                frame "Kg", Default {
                  n326 = Multiply(x=w830, y=1000.0) -> (x*y=w833:dbl)
                  n327 = Quotient & Remainder(x=w833, y=2.0) -> (x-y*floor(x/y)=w834:dbl)  [unwired: 1 out]
                  n328 = Subtract(x=w833, y=w834) -> (x-y=w832:dbl)
                  n329 = Divide(x=w832, y=1000.0) -> (x/y=w827:dbl)
                  n330 = Absolute Value(x=w827) -> (abs(x)=w825:dbl)
                  n331 = Greater?(x=w825, y=0.004) -> (0:w828:bool)
                  n332 = case shown="False" w828 {
                    tunnel: w827 -> [_ w839]
                    tunnel: [0.0 w839] -> w826
                    frame False {
                    }
                    frame True {
                    }
                  }
                }
                frame "N" {
                  n333 = Multiply(x=w845, y=100.0) -> (x*y=w848:dbl)
                  n334 = Quotient & Remainder(x=w848, y=2.0) -> (x-y*floor(x/y)=w849:dbl)  [unwired: 1 out]
                  n335 = Subtract(x=w848, y=w849) -> (x-y=w847:dbl)
                  n336 = Divide(x=w847, y=100.0) -> (x/y=w843:dbl)
                  n337 = Absolute Value(x=w843) -> (abs(x)=w840:dbl)
                  n338 = Greater?(x=w840, y=0.04) -> (0:w844:bool)
                  n339 = case shown="False" w844 {
                    tunnel: w843 -> [_ w854]
                    tunnel: [0.0 w854] -> w842
                    frame False {
                    }
                    frame True {
                    }
                  }
                }
                frame "g" {
                  n340 = Multiply(x=w860, y=1.0) -> (x*y=w863:dbl)
                  n341 = Quotient & Remainder(x=w863, y=2.0) -> (x-y*floor(x/y)=w864:dbl)  [unwired: 1 out]
                  n342 = Subtract(x=w863, y=w864) -> (x-y=w862:dbl)
                  n343 = Divide(x=w862, y=1.0) -> (x/y=w858:dbl)
                  n344 = Absolute Value(x=w858) -> (abs(x)=w855:dbl)
                  n345 = Greater?(x=w855, y=4.0) -> (0:w859:bool)
                  n346 = case shown="False" w859 {
                    tunnel: w858 -> [_ w869]
                    tunnel: [0.0 w869] -> w857
                    frame False {
                    }
                    frame True {
                    }
                  }
                }
                frame "daN" {
                  n347 = Multiply(x=w875, y=1000.0) -> (x*y=w878:dbl)
                  n348 = Quotient & Remainder(x=w878, y=2.0) -> (x-y*floor(x/y)=w879:dbl)  [unwired: 1 out]
                  n349 = Subtract(x=w878, y=w879) -> (x-y=w877:dbl)
                  n350 = Divide(x=w877, y=1000.0) -> (x/y=w873:dbl)
                  n351 = Absolute Value(x=w873) -> (abs(x)=w870:dbl)
                  n352 = Greater?(x=w870, y=0.004) -> (0:w874:bool)
                  n353 = case shown="False" w874 {
                    tunnel: w873 -> [_ w884]
                    tunnel: [0.0 w884] -> w872
                    frame False {
                    }
                    frame True {
                    }
                  }
                }
                frame "cN" {
                  n354 = Multiply(x=w890, y=1.0) -> (x*y=w893:dbl)
                  n355 = Quotient & Remainder(x=w893, y=2.0) -> (x-y*floor(x/y)=w894:dbl)  [unwired: 1 out]
                  n356 = Subtract(x=w893, y=w894) -> (x-y=w892:dbl)
                  n357 = Divide(x=w892, y=1.0) -> (x/y=w888:dbl)
                  n358 = Absolute Value(x=w888) -> (abs(x)=w885:dbl)
                  n359 = Greater?(x=w885, y=4.0) -> (0:w889:bool)
                  n360 = case shown="False" w889 {
                    tunnel: w888 -> [_ w899]
                    tunnel: [0.0 w899] -> w887
                    frame False {
                    }
                    frame True {
                    }
                  }
                }
                frame "KN" {
                }
                frame "lb" {
                  n361 = Multiply(x=w907, y=1000.0) -> (x*y=w910:dbl)
                  n362 = Quotient & Remainder(x=w910, y=5.0) -> (x-y*floor(x/y)=w911:dbl)  [unwired: 1 out]
                  n363 = Subtract(x=w910, y=w911) -> (x-y=w909:dbl)
                  n364 = Divide(x=w909, y=1000.0) -> (x/y=w905:dbl)
                  n365 = Absolute Value(x=w905) -> (abs(x)=w902:dbl)
                  n366 = Greater?(x=w902, y=0.01) -> (0:w906:bool)
                  n367 = case shown="False" w906 {
                    tunnel: w905 -> [_ w916]
                    tunnel: [0.0 w916] -> w904
                    frame False {
                    }
                    frame True {
                    }
                  }
                }
              }
            }
            frame 1 {
              n368 = case shown="\"lb\"" w917 {
                tunnel: [w921 w923 w925 w934 w936 w945 w948] -> w920
                tunnel: [2 1 0 0 0 0 3] -> w919
                tunnel: w918 -> [w921 w923 w926 w934 w937 w945 w947]
                frame "Kg", Default {
                }
                frame "N" {
                }
                frame "g" {
                  n369 = Multiply(x=w926, y=1.0) -> (x*y=w929:dbl)
                  n370 = Quotient & Remainder(x=w929, y=10.0) -> (x-y*floor(x/y)=w930:dbl)  [unwired: 1 out]
                  n371 = Subtract(x=w929, y=w930) -> (x-y=w928:dbl)
                  n372 = Divide(x=w928, y=1.0) -> (x/y=w925:dbl)
                }
                frame "daN" {
                }
                frame "cN" {
                  n373 = Multiply(x=w937, y=1.0) -> (x*y=w940:dbl)
                  n374 = Quotient & Remainder(x=w940, y=10.0) -> (x-y*floor(x/y)=w941:dbl)  [unwired: 1 out]
                  n375 = Subtract(x=w940, y=w941) -> (x-y=w939:dbl)
                  n376 = Divide(x=w939, y=1.0) -> (x/y=w936:dbl)
                }
                frame "KN" {
                }
                frame "lb" {
                  n377 = Multiply(x=w947, y=200.0) -> (x*y=w951:dbl)
                  n378 = Quotient & Remainder(x=w951, y=5.0) -> (x-y*floor(x/y)=w952:dbl)  [unwired: 1 out]
                  n379 = Subtract(x=w951, y=w952) -> (x-y=w950:dbl)
                  n380 = Divide(x=w950, y=200.0) -> (x/y=w948:dbl)
                }
              }
            }
          }
        }
        frame 6 {
          n381 = case shown="0, Default" w958 {
            tunnel: w959 -> [w964 w1053]
            tunnel: [w963 w1052] -> w957
            tunnel: [w962 w1051] -> w956
            tunnel: w960 -> [w961 w1050]
            frame 0, Default {
              n382 = case shown="\"Kg\", Default" w964 {
                tunnel: [w967 w982 w997 w1012 w1027 w1040 w1044] -> w963
                tunnel: [3 2 0 3 0 0 2] -> w962
                tunnel: w961 -> [w970 w985 w1000 w1015 w1030 w1040 w1045]
                frame "Kg", Default {
                  n383 = Multiply(x=w970, y=1000.0) -> (x*y=w973:dbl)
                  n384 = Quotient & Remainder(x=w973, y=5.0) -> (x-y*floor(x/y)=w974:dbl)  [unwired: 1 out]
                  n385 = Subtract(x=w973, y=w974) -> (x-y=w972:dbl)
                  n386 = Divide(x=w972, y=1000.0) -> (x/y=w968:dbl)
                  n387 = Absolute Value(x=w968) -> (abs(x)=w965:dbl)
                  n388 = Greater?(x=w965, y=0.01) -> (0:w969:bool)
                  n389 = case shown="False" w969 {
                    tunnel: w968 -> [_ w979]
                    tunnel: [0.0 w979] -> w967
                    frame False {
                    }
                    frame True {
                    }
                  }
                }
                frame "N" {
                  n390 = Multiply(x=w985, y=100.0) -> (x*y=w988:dbl)
                  n391 = Quotient & Remainder(x=w988, y=5.0) -> (x-y*floor(x/y)=w989:dbl)  [unwired: 1 out]
                  n392 = Subtract(x=w988, y=w989) -> (x-y=w987:dbl)
                  n393 = Divide(x=w987, y=100.0) -> (x/y=w983:dbl)
                  n394 = Absolute Value(x=w983) -> (abs(x)=w980:dbl)
                  n395 = Greater?(x=w980, y=0.1) -> (0:w984:bool)
                  n396 = case shown="False" w984 {
                    tunnel: w983 -> [_ w994]
                    tunnel: [0.0 w994] -> w982
                    frame False {
                    }
                    frame True {
                    }
                  }
                }
                frame "g" {
                  n397 = Multiply(x=w1000, y=1.0) -> (x*y=w1003:dbl)
                  n398 = Quotient & Remainder(x=w1003, y=5.0) -> (x-y*floor(x/y)=w1004:dbl)  [unwired: 1 out]
                  n399 = Subtract(x=w1003, y=w1004) -> (x-y=w1002:dbl)
                  n400 = Divide(x=w1002, y=1.0) -> (x/y=w998:dbl)
                  n401 = Absolute Value(x=w998) -> (abs(x)=w995:dbl)
                  n402 = Greater?(x=w995, y=10.0) -> (0:w999:bool)
                  n403 = case shown="False" w999 {
                    tunnel: w998 -> [_ w1009]
                    tunnel: [0.0 w1009] -> w997
                    frame False {
                    }
                    frame True {
                    }
                  }
                }
                frame "daN" {
                  n404 = Multiply(x=w1015, y=1000.0) -> (x*y=w1018:dbl)
                  n405 = Quotient & Remainder(x=w1018, y=5.0) -> (x-y*floor(x/y)=w1019:dbl)  [unwired: 1 out]
                  n406 = Subtract(x=w1018, y=w1019) -> (x-y=w1017:dbl)
                  n407 = Divide(x=w1017, y=1000.0) -> (x/y=w1013:dbl)
                  n408 = Absolute Value(x=w1013) -> (abs(x)=w1010:dbl)
                  n409 = Greater?(x=w1010, y=0.01) -> (0:w1014:bool)
                  n410 = case shown="False" w1014 {
                    tunnel: w1013 -> [_ w1024]
                    tunnel: [0.0 w1024] -> w1012
                    frame False {
                    }
                    frame True {
                    }
                  }
                }
                frame "cN" {
                  n411 = Multiply(x=w1030, y=1.0) -> (x*y=w1034:dbl)
                  n412 = Quotient & Remainder(x=w1034, y=5.0) -> (x-y*floor(x/y)=w1035:dbl)  [unwired: 1 out]
                  n413 = Subtract(x=w1034, y=w1035) -> (x-y=w1033:dbl)
                  n414 = Divide(x=w1033, y=1.0) -> (x/y=w1028:dbl)
                  n415 = Absolute Value(x=w1028) -> (abs(x)=w1025:dbl)
                  n416 = Greater?(x=w1025, y=10.0) -> (0:w1029:bool)
                  n417 = case shown="False" w1029 {
                    tunnel: w1028 -> [_ w1039]
                    tunnel: [0.0 w1039] -> w1027
                    frame False {
                    }
                    frame True {
                    }
                  }
                }
                frame "KN" {
                }
                frame "lb" {
                  n418 = Absolute Value(x=w1045) -> (abs(x)=w1042:dbl)
                  n419 = Greater?(x=w1042, y=0.02) -> (0:w1046:bool)
                  n420 = case shown="False" w1046 {
                    tunnel: w1045 -> [_ w1049]
                    tunnel: [0.0 w1049] -> w1044
                    frame False {
                    }
                    frame True {
                    }
                  }
                }
              }
            }
            frame 1 {
              n421 = case shown="\"lb\"" w1053 {
                tunnel: [w1055 w1064 w1073 w1082 w1092 w1099 w1102] -> w1052
                tunnel: [3 2 0 3 0 0 2] -> w1051
                tunnel: w1050 -> [w1054 w1063 w1072 w1081 w1090 w1099 w1101]
                frame "Kg", Default {
                  n422 = Multiply(x=w1054, y=200.0) -> (x*y=w1058:dbl)
                  n423 = Quotient & Remainder(x=w1058, y=5.0) -> (x-y*floor(x/y)=w1059:dbl)  [unwired: 1 out]
                  n424 = Subtract(x=w1058, y=w1059) -> (x-y=w1057:dbl)
                  n425 = Divide(x=w1057, y=200.0) -> (x/y=w1055:dbl)
                }
                frame "N" {
                  n426 = Multiply(x=w1063, y=20.0) -> (x*y=w1067:dbl)
                  n427 = Quotient & Remainder(x=w1067, y=5.0) -> (x-y*floor(x/y)=w1068:dbl)  [unwired: 1 out]
                  n428 = Subtract(x=w1067, y=w1068) -> (x-y=w1066:dbl)
                  n429 = Divide(x=w1066, y=20.0) -> (x/y=w1064:dbl)
                }
                frame "g" {
                  n430 = Multiply(x=w1072, y=20.0) -> (x*y=w1076:dbl)
                  n431 = Quotient & Remainder(x=w1076, y=5.0) -> (x-y*floor(x/y)=w1077:dbl)  [unwired: 1 out]
                  n432 = Subtract(x=w1076, y=w1077) -> (x-y=w1075:dbl)
                  n433 = Divide(x=w1075, y=20.0) -> (x/y=w1073:dbl)
                }
                frame "daN" {
                  n434 = Multiply(x=w1081, y=200.0) -> (x*y=w1085:dbl)
                  n435 = Quotient & Remainder(x=w1085, y=5.0) -> (x-y*floor(x/y)=w1086:dbl)  [unwired: 1 out]
                  n436 = Subtract(x=w1085, y=w1086) -> (x-y=w1084:dbl)
                  n437 = Divide(x=w1084, y=200.0) -> (x/y=w1082:dbl)
                }
                frame "cN" {
                  n438 = Multiply(x=w1090, y=20.0) -> (x*y=w1095:dbl)
                  n439 = Quotient & Remainder(x=w1095, y=5.0) -> (x-y*floor(x/y)=w1096:dbl)  [unwired: 1 out]
                  n440 = Subtract(x=w1095, y=w1096) -> (x-y=w1094:dbl)
                  n441 = Divide(x=w1094, y=20.0) -> (x/y=w1092:dbl)
                }
                frame "KN" {
                }
                frame "lb" {
                  n442 = Multiply(x=w1101, y=100.0) -> (x*y=w1105:dbl)
                  n443 = Quotient & Remainder(x=w1105, y=5.0) -> (x-y*floor(x/y)=w1106:dbl)  [unwired: 1 out]
                  n444 = Subtract(x=w1105, y=w1106) -> (x-y=w1104:dbl)
                  n445 = Divide(x=w1104, y=100.0) -> (x/y=w1102:dbl)
                }
              }
            }
          }
        }
        frame 7 {
          n446 = case shown="0, Default" w1112 {
            tunnel: [w1118 w1179] -> w1111
            tunnel: [w1117 w1178] -> w1110
            tunnel: w1114 -> [w1116 w1177]
            tunnel: w1113 -> [w1115 w1176]
            frame 0, Default {
              n447 = case shown="\"Kg\", Default" w1115 {
                tunnel: [w1121 w1129 w1137 w1144 w1152 w1159 w1163] -> w1118
                tunnel: [2 1 0 2 0 0 2] -> w1117
                tunnel: w1116 -> [w1122 w1130 w1138 w1146 w1154 w1159 w1166]
                frame "Kg", Default {
                  n448 = Absolute Value(x=w1122) -> (abs(x)=w1119:dbl)
                  n449 = Greater?(x=w1119, y=0.02) -> (0:w1123:bool)
                  n450 = case shown="False" w1123 {
                    tunnel: w1122 -> [_ w1126]
                    tunnel: [0.0 w1126] -> w1121
                    frame False {
                    }
                    frame True {
                    }
                  }
                }
                frame "N" {
                  n451 = Absolute Value(x=w1130) -> (abs(x)=w1127:dbl)
                  n452 = Greater?(x=w1127, y=0.2) -> (0:w1131:bool)
                  n453 = case shown="False" w1131 {
                    tunnel: w1130 -> [_ w1134]
                    tunnel: [0.0 w1134] -> w1129
                    frame False {
                    }
                    frame True {
                    }
                  }
                }
                frame "g" {
                  n454 = Absolute Value(x=w1138) -> (abs(x)=w1135:dbl)
                  n455 = Greater?(x=w1135, y=2.0) -> (0:w1139:bool)
                  n456 = case shown="False" w1139 {
                    tunnel: w1138 -> [_ w1142]
                    tunnel: [0.0 w1142] -> w1137
                    frame False {
                    }
                    frame True {
                    }
                  }
                }
                frame "daN" {
                  n457 = Absolute Value(x=w1146) -> (abs(x)=w1143:dbl)
                  n458 = Greater?(x=w1143, y=0.02) -> (0:w1147:bool)
                  n459 = case shown="False" w1147 {
                    tunnel: w1146 -> [_ w1150]
                    tunnel: [0.0 w1150] -> w1144
                    frame False {
                    }
                    frame True {
                    }
                  }
                }
                frame "cN" {
                  n460 = Absolute Value(x=w1154) -> (abs(x)=w1151:dbl)
                  n461 = Greater?(x=w1151, y=2.0) -> (0:w1155:bool)
                  n462 = case shown="False" w1155 {
                    tunnel: w1154 -> [_ w1158]
                    tunnel: [0.0 w1158] -> w1152
                    frame False {
                    }
                    frame True {
                    }
                  }
                }
                frame "KN" {
                }
                frame "lb" {
                  n463 = Multiply(x=w1166, y=100.0) -> (x*y=w1169:dbl)
                  n464 = Quotient & Remainder(x=w1169, y=2.0) -> (x-y*floor(x/y)=w1170:dbl)  [unwired: 1 out]
                  n465 = Subtract(x=w1169, y=w1170) -> (x-y=w1168:dbl)
                  n466 = Divide(x=w1168, y=100.0) -> (x/y=w1164:dbl)
                  n467 = Absolute Value(x=w1164) -> (abs(x)=w1161:dbl)
                  n468 = Greater?(x=w1161, y=0.04) -> (0:w1165:bool)
                  n469 = case shown="False" w1165 {
                    tunnel: w1164 -> [_ w1175]
                    tunnel: [0.0 w1175] -> w1163
                    frame False {
                    }
                    frame True {
                    }
                  }
                }
              }
            }
            frame 1 {
              n470 = case shown="\"lb\"" w1176 {
                tunnel: [w1181 w1189 w1198 w1200 w1209 w1211 w1213] -> w1179
                tunnel: [2 1 0 2 0 0 1] -> w1178
                tunnel: w1177 -> [w1180 w1190 w1198 w1201 w1209 w1211 w1213]
                frame "Kg", Default {
                  n471 = Multiply(x=w1180, y=100.0) -> (x*y=w1184:dbl)
                  n472 = Quotient & Remainder(x=w1184, y=5.0) -> (x-y*floor(x/y)=w1185:dbl)  [unwired: 1 out]
                  n473 = Subtract(x=w1184, y=w1185) -> (x-y=w1183:dbl)
                  n474 = Divide(x=w1183, y=100.0) -> (x/y=w1181:dbl)
                }
                frame "N" {
                  n475 = Multiply(x=w1190, y=10.0) -> (x*y=w1193:dbl)
                  n476 = Quotient & Remainder(x=w1193, y=5.0) -> (x-y*floor(x/y)=w1194:dbl)  [unwired: 1 out]
                  n477 = Subtract(x=w1193, y=w1194) -> (x-y=w1192:dbl)
                  n478 = Divide(x=w1192, y=10.0) -> (x/y=w1189:dbl)
                }
                frame "g" {
                }
                frame "daN" {
                  n479 = Multiply(x=w1201, y=100.0) -> (x*y=w1204:dbl)
                  n480 = Quotient & Remainder(x=w1204, y=5.0) -> (x-y*floor(x/y)=w1205:dbl)  [unwired: 1 out]
                  n481 = Subtract(x=w1204, y=w1205) -> (x-y=w1203:dbl)
                  n482 = Divide(x=w1203, y=100.0) -> (x/y=w1200:dbl)
                }
                frame "cN" {
                }
                frame "KN" {
                }
                frame "lb" {
                }
              }
            }
          }
        }
        frame 18 {
          n483 = case shown="1" w1217 {
            tunnel: [w1223 w1284] -> w1216
            tunnel: [w1222 w1283] -> w1215
            tunnel: w1219 -> [w1221 w1282]
            tunnel: w1218 -> [w1220 w1281]
            frame 0, Default {
              n484 = case shown="\"Kg\", Default" w1220 {
                tunnel: [w1226 w1234 w1242 w1249 w1257 w1264 w1268] -> w1223
                tunnel: [2 1 0 2 0 0 2] -> w1222
                tunnel: w1221 -> [w1227 w1235 w1243 w1251 w1259 w1264 w1271]
                frame "Kg", Default {
                  n485 = Absolute Value(x=w1227) -> (abs(x)=w1224:dbl)
                  n486 = Greater?(x=w1224, y=0.02) -> (0:w1228:bool)
                  n487 = case shown="False" w1228 {
                    tunnel: w1227 -> [_ w1231]
                    tunnel: [0.0 w1231] -> w1226
                    frame False {
                    }
                    frame True {
                    }
                  }
                }
                frame "N" {
                  n488 = Absolute Value(x=w1235) -> (abs(x)=w1232:dbl)
                  n489 = Greater?(x=w1232, y=0.2) -> (0:w1236:bool)
                  n490 = case shown="False" w1236 {
                    tunnel: w1235 -> [_ w1239]
                    tunnel: [0.0 w1239] -> w1234
                    frame False {
                    }
                    frame True {
                    }
                  }
                }
                frame "g" {
                  n491 = Absolute Value(x=w1243) -> (abs(x)=w1240:dbl)
                  n492 = Greater?(x=w1240, y=2.0) -> (0:w1244:bool)
                  n493 = case shown="False" w1244 {
                    tunnel: w1243 -> [_ w1247]
                    tunnel: [0.0 w1247] -> w1242
                    frame False {
                    }
                    frame True {
                    }
                  }
                }
                frame "daN" {
                  n494 = Absolute Value(x=w1251) -> (abs(x)=w1248:dbl)
                  n495 = Greater?(x=w1248, y=0.02) -> (0:w1252:bool)
                  n496 = case shown="False" w1252 {
                    tunnel: w1251 -> [_ w1255]
                    tunnel: [0.0 w1255] -> w1249
                    frame False {
                    }
                    frame True {
                    }
                  }
                }
                frame "cN" {
                  n497 = Absolute Value(x=w1259) -> (abs(x)=w1256:dbl)
                  n498 = Greater?(x=w1256, y=2.0) -> (0:w1260:bool)
                  n499 = case shown="False" w1260 {
                    tunnel: w1259 -> [_ w1263]
                    tunnel: [0.0 w1263] -> w1257
                    frame False {
                    }
                    frame True {
                    }
                  }
                }
                frame "KN" {
                }
                frame "lb" {
                  n500 = Multiply(x=w1271, y=100.0) -> (x*y=w1274:dbl)
                  n501 = Quotient & Remainder(x=w1274, y=2.0) -> (x-y*floor(x/y)=w1275:dbl)  [unwired: 1 out]
                  n502 = Subtract(x=w1274, y=w1275) -> (x-y=w1273:dbl)
                  n503 = Divide(x=w1273, y=100.0) -> (x/y=w1269:dbl)
                  n504 = Absolute Value(x=w1269) -> (abs(x)=w1266:dbl)
                  n505 = Greater?(x=w1266, y=0.04) -> (0:w1270:bool)
                  n506 = case shown="False" w1270 {
                    tunnel: w1269 -> [_ w1280]
                    tunnel: [0.0 w1280] -> w1268
                    frame False {
                    }
                    frame True {
                    }
                  }
                }
              }
            }
            frame 1 {
              n507 = case shown="\"Kg\", Default" w1281 {
                tunnel: [w1287 w1295 w1303 w1310 w1318 w1325 w1329] -> w1284
                tunnel: [2 1 0 2 0 0 2] -> w1283
                tunnel: w1282 -> [w1288 w1296 w1304 w1312 w1320 w1325 w1332]
                frame "Kg", Default {
                  n508 = Absolute Value(x=w1288) -> (abs(x)=w1285:dbl)
                  n509 = Greater?(x=w1285, y=0.02) -> (0:w1289:bool)
                  n510 = case shown="False" w1289 {
                    tunnel: w1288 -> [_ w1292]
                    tunnel: [0.0 w1292] -> w1287
                    frame False {
                    }
                    frame True {
                    }
                  }
                }
                frame "N" {
                  n511 = Absolute Value(x=w1296) -> (abs(x)=w1293:dbl)
                  n512 = Greater?(x=w1293, y=0.2) -> (0:w1297:bool)
                  n513 = case shown="False" w1297 {
                    tunnel: w1296 -> [_ w1300]
                    tunnel: [0.0 w1300] -> w1295
                    frame False {
                    }
                    frame True {
                    }
                  }
                }
                frame "g" {
                  n514 = Absolute Value(x=w1304) -> (abs(x)=w1301:dbl)
                  n515 = Greater?(x=w1301, y=2.0) -> (0:w1305:bool)
                  n516 = case shown="False" w1305 {
                    tunnel: w1304 -> [_ w1308]
                    tunnel: [0.0 w1308] -> w1303
                    frame False {
                    }
                    frame True {
                    }
                  }
                }
                frame "daN" {
                  n517 = Absolute Value(x=w1312) -> (abs(x)=w1309:dbl)
                  n518 = Greater?(x=w1309, y=0.02) -> (0:w1313:bool)
                  n519 = case shown="False" w1313 {
                    tunnel: w1312 -> [_ w1316]
                    tunnel: [0.0 w1316] -> w1310
                    frame False {
                    }
                    frame True {
                    }
                  }
                }
                frame "cN" {
                  n520 = Absolute Value(x=w1320) -> (abs(x)=w1317:dbl)
                  n521 = Greater?(x=w1317, y=2.0) -> (0:w1321:bool)
                  n522 = case shown="False" w1321 {
                    tunnel: w1320 -> [_ w1324]
                    tunnel: [0.0 w1324] -> w1318
                    frame False {
                    }
                    frame True {
                    }
                  }
                }
                frame "KN" {
                }
                frame "lb" {
                  n523 = Multiply(x=w1332, y=100.0) -> (x*y=w1335:dbl)
                  n524 = Quotient & Remainder(x=w1335, y=2.0) -> (x-y*floor(x/y)=w1336:dbl)  [unwired: 1 out]
                  n525 = Subtract(x=w1335, y=w1336) -> (x-y=w1334:dbl)
                  n526 = Divide(x=w1334, y=100.0) -> (x/y=w1330:dbl)
                  n527 = Absolute Value(x=w1330) -> (abs(x)=w1327:dbl)
                  n528 = Greater?(x=w1327, y=0.04) -> (0:w1331:bool)
                  n529 = case shown="False" w1331 {
                    tunnel: w1330 -> [_ w1341]
                    tunnel: [0.0 w1341] -> w1329
                    frame False {
                    }
                    frame True {
                    }
                  }
                }
              }
            }
          }
        }
        frame 22 {
          n530 = case shown="1" w1344 {
            tunnel: [w1350 w1411] -> w1343
            tunnel: [w1349 w1410] -> w1342
            tunnel: w1346 -> [w1348 w1409]
            tunnel: w1345 -> [w1347 w1408]
            frame 0, Default {
              n531 = case shown="\"Kg\", Default" w1347 {
                tunnel: [w1353 w1361 w1369 w1376 w1384 w1391 w1395] -> w1350
                tunnel: [2 1 0 2 0 0 2] -> w1349
                tunnel: w1348 -> [w1354 w1362 w1370 w1378 w1386 w1391 w1398]
                frame "Kg", Default {
                  n532 = Absolute Value(x=w1354) -> (abs(x)=w1351:dbl)
                  n533 = Greater?(x=w1351, y=0.02) -> (0:w1355:bool)
                  n534 = case shown="False" w1355 {
                    tunnel: w1354 -> [_ w1358]
                    tunnel: [0.0 w1358] -> w1353
                    frame False {
                    }
                    frame True {
                    }
                  }
                }
                frame "N" {
                  n535 = Absolute Value(x=w1362) -> (abs(x)=w1359:dbl)
                  n536 = Greater?(x=w1359, y=0.2) -> (0:w1363:bool)
                  n537 = case shown="False" w1363 {
                    tunnel: w1362 -> [_ w1366]
                    tunnel: [0.0 w1366] -> w1361
                    frame False {
                    }
                    frame True {
                    }
                  }
                }
                frame "g" {
                  n538 = Absolute Value(x=w1370) -> (abs(x)=w1367:dbl)
                  n539 = Greater?(x=w1367, y=2.0) -> (0:w1371:bool)
                  n540 = case shown="False" w1371 {
                    tunnel: w1370 -> [_ w1374]
                    tunnel: [0.0 w1374] -> w1369
                    frame False {
                    }
                    frame True {
                    }
                  }
                }
                frame "daN" {
                  n541 = Absolute Value(x=w1378) -> (abs(x)=w1375:dbl)
                  n542 = Greater?(x=w1375, y=0.02) -> (0:w1379:bool)
                  n543 = case shown="False" w1379 {
                    tunnel: w1378 -> [_ w1382]
                    tunnel: [0.0 w1382] -> w1376
                    frame False {
                    }
                    frame True {
                    }
                  }
                }
                frame "cN" {
                  n544 = Absolute Value(x=w1386) -> (abs(x)=w1383:dbl)
                  n545 = Greater?(x=w1383, y=2.0) -> (0:w1387:bool)
                  n546 = case shown="False" w1387 {
                    tunnel: w1386 -> [_ w1390]
                    tunnel: [0.0 w1390] -> w1384
                    frame False {
                    }
                    frame True {
                    }
                  }
                }
                frame "KN" {
                }
                frame "lb" {
                  n547 = Multiply(x=w1398, y=100.0) -> (x*y=w1401:dbl)
                  n548 = Quotient & Remainder(x=w1401, y=2.0) -> (x-y*floor(x/y)=w1402:dbl)  [unwired: 1 out]
                  n549 = Subtract(x=w1401, y=w1402) -> (x-y=w1400:dbl)
                  n550 = Divide(x=w1400, y=100.0) -> (x/y=w1396:dbl)
                  n551 = Absolute Value(x=w1396) -> (abs(x)=w1393:dbl)
                  n552 = Greater?(x=w1393, y=0.04) -> (0:w1397:bool)
                  n553 = case shown="False" w1397 {
                    tunnel: w1396 -> [_ w1407]
                    tunnel: [0.0 w1407] -> w1395
                    frame False {
                    }
                    frame True {
                    }
                  }
                }
              }
            }
            frame 1 {
              n554 = case shown="\"Kg\", Default" w1408 {
                tunnel: [w1414 w1422 w1430 w1437 w1445 w1452 w1456] -> w1411
                tunnel: [2 1 0 2 0 0 2] -> w1410
                tunnel: w1409 -> [w1415 w1423 w1431 w1439 w1447 w1452 w1459]
                frame "Kg", Default {
                  n555 = Absolute Value(x=w1415) -> (abs(x)=w1412:dbl)
                  n556 = Greater?(x=w1412, y=0.02) -> (0:w1416:bool)
                  n557 = case shown="False" w1416 {
                    tunnel: w1415 -> [_ w1419]
                    tunnel: [0.0 w1419] -> w1414
                    frame False {
                    }
                    frame True {
                    }
                  }
                }
                frame "N" {
                  n558 = Absolute Value(x=w1423) -> (abs(x)=w1420:dbl)
                  n559 = Greater?(x=w1420, y=0.2) -> (0:w1424:bool)
                  n560 = case shown="False" w1424 {
                    tunnel: w1423 -> [_ w1427]
                    tunnel: [0.0 w1427] -> w1422
                    frame False {
                    }
                    frame True {
                    }
                  }
                }
                frame "g" {
                  n561 = Absolute Value(x=w1431) -> (abs(x)=w1428:dbl)
                  n562 = Greater?(x=w1428, y=2.0) -> (0:w1432:bool)
                  n563 = case shown="False" w1432 {
                    tunnel: w1431 -> [_ w1435]
                    tunnel: [0.0 w1435] -> w1430
                    frame False {
                    }
                    frame True {
                    }
                  }
                }
                frame "daN" {
                  n564 = Absolute Value(x=w1439) -> (abs(x)=w1436:dbl)
                  n565 = Greater?(x=w1436, y=0.02) -> (0:w1440:bool)
                  n566 = case shown="False" w1440 {
                    tunnel: w1439 -> [_ w1443]
                    tunnel: [0.0 w1443] -> w1437
                    frame False {
                    }
                    frame True {
                    }
                  }
                }
                frame "cN" {
                  n567 = Absolute Value(x=w1447) -> (abs(x)=w1444:dbl)
                  n568 = Greater?(x=w1444, y=2.0) -> (0:w1448:bool)
                  n569 = case shown="False" w1448 {
                    tunnel: w1447 -> [_ w1451]
                    tunnel: [0.0 w1451] -> w1445
                    frame False {
                    }
                    frame True {
                    }
                  }
                }
                frame "KN" {
                }
                frame "lb" {
                  n570 = Multiply(x=w1459, y=100.0) -> (x*y=w1462:dbl)
                  n571 = Quotient & Remainder(x=w1462, y=2.0) -> (x-y*floor(x/y)=w1463:dbl)  [unwired: 1 out]
                  n572 = Subtract(x=w1462, y=w1463) -> (x-y=w1461:dbl)
                  n573 = Divide(x=w1461, y=100.0) -> (x/y=w1457:dbl)
                  n574 = Absolute Value(x=w1457) -> (abs(x)=w1454:dbl)
                  n575 = Greater?(x=w1454, y=0.04) -> (0:w1458:bool)
                  n576 = case shown="False" w1458 {
                    tunnel: w1457 -> [_ w1468]
                    tunnel: [0.0 w1468] -> w1456
                    frame False {
                    }
                    frame True {
                    }
                  }
                }
              }
            }
          }
        }
        frame 8 {
          n577 = case shown="0, Default" w1471 {
            tunnel: [w1477 w1559] -> w1470
            tunnel: [w1476 w1558] -> w1469
            tunnel: w1473 -> [w1475 w1557]
            tunnel: w1472 -> [w1474 w1556]
            frame 0, Default {
              n578 = case shown="\"lb\"" w1474 {
                tunnel: [w1480 w1495 w1509 w1517 w1532 w1539 w1543] -> w1477
                tunnel: [2 1 0 2 0 0 2] -> w1476
                tunnel: w1475 -> [w1483 w1498 w1510 w1522 w1533 w1539 w1546]
                frame "Kg", Default {
                  n579 = Multiply(x=w1483, y=100.0) -> (x*y=w1486:dbl)
                  n580 = Quotient & Remainder(x=w1486, y=2.0) -> (x-y*floor(x/y)=w1487:dbl)  [unwired: 1 out]
                  n581 = Subtract(x=w1486, y=w1487) -> (x-y=w1485:dbl)
                  n582 = Divide(x=w1485, y=100.0) -> (x/y=w1481:dbl)
                  n583 = Absolute Value(x=w1481) -> (abs(x)=w1478:dbl)
                  n584 = Greater?(x=w1478, y=0.04) -> (0:w1482:bool)
                  n585 = case shown="False" w1482 {
                    tunnel: w1481 -> [_ w1492]
                    tunnel: [0.0 w1492] -> w1480
                    frame False {
                    }
                    frame True {
                    }
                  }
                }
                frame "N" {
                  n586 = Multiply(x=w1498, y=10.0) -> (x*y=w1501:dbl)
                  n587 = Quotient & Remainder(x=w1501, y=2.0) -> (x-y*floor(x/y)=w1502:dbl)  [unwired: 1 out]
                  n588 = Subtract(x=w1501, y=w1502) -> (x-y=w1500:dbl)
                  n589 = Divide(x=w1500, y=10.0) -> (x/y=w1494:dbl)
                  n590 = Absolute Value(x=w1494) -> (abs(x)=w1493:dbl)
                  n591 = Greater?(x=w1493, y=0.4) -> (0:w1497:bool)
                  n592 = case shown="False" w1497 {
                    tunnel: w1494 -> [_ w1507]
                    tunnel: [0.0 w1507] -> w1495
                    frame False {
                    }
                    frame True {
                    }
                  }
                }
                frame "g" {
                  n593 = Absolute Value(x=w1510) -> (abs(x)=w1508:dbl)
                  n594 = Greater?(x=w1508, y=2.0) -> (0:w1512:bool)
                  n595 = case shown="False" w1512 {
                    tunnel: w1510 -> [_ w1515]
                    tunnel: [0.0 w1515] -> w1509
                    frame False {
                    }
                    frame True {
                    }
                  }
                }
                frame "daN" {
                  n596 = Multiply(x=w1522, y=100.0) -> (x*y=w1525:dbl)
                  n597 = Quotient & Remainder(x=w1525, y=2.0) -> (x-y*floor(x/y)=w1526:dbl)  [unwired: 1 out]
                  n598 = Subtract(x=w1525, y=w1526) -> (x-y=w1524:dbl)
                  n599 = Divide(x=w1524, y=100.0) -> (x/y=w1518:dbl)
                  n600 = Absolute Value(x=w1518) -> (abs(x)=w1516:dbl)
                  n601 = Greater?(x=w1516, y=0.04) -> (0:w1520:bool)
                  n602 = case shown="False" w1520 {
                    tunnel: w1518 -> [_ w1530]
                    tunnel: [0.0 w1530] -> w1517
                    frame False {
                    }
                    frame True {
                    }
                  }
                }
                frame "cN" {
                  n603 = Absolute Value(x=w1533) -> (abs(x)=w1531:dbl)
                  n604 = Greater?(x=w1531, y=2.0) -> (0:w1535:bool)
                  n605 = case shown="False" w1535 {
                    tunnel: w1533 -> [_ w1538]
                    tunnel: [0.0 w1538] -> w1532
                    frame False {
                    }
                    frame True {
                    }
                  }
                }
                frame "KN" {
                }
                frame "lb" {
                  n606 = Multiply(x=w1546, y=100.0) -> (x*y=w1549:dbl)
                  n607 = Quotient & Remainder(x=w1549, y=5.0) -> (x-y*floor(x/y)=w1550:dbl)  [unwired: 1 out]
                  n608 = Subtract(x=w1549, y=w1550) -> (x-y=w1548:dbl)
                  n609 = Divide(x=w1548, y=100.0) -> (x/y=w1542:dbl)
                  n610 = Absolute Value(x=w1542) -> (abs(x)=w1541:dbl)
                  n611 = Greater?(x=w1541, y=0.1) -> (0:w1545:bool)
                  n612 = case shown="False" w1545 {
                    tunnel: w1542 -> [_ w1555]
                    tunnel: [0.0 w1555] -> w1543
                    frame False {
                    }
                    frame True {
                    }
                  }
                }
              }
            }
            frame 1 {
              n613 = case shown="\"Kg\", Default" w1556 {
                tunnel: [w1560 w1569 w1578 w1581 w1589 w1591 w1594] -> w1559
                tunnel: [1 0 0 1 0 0 1] -> w1558
                tunnel: w1557 -> [w1561 w1570 w1578 w1580 w1589 w1591 w1593]
                frame "Kg", Default {
                  n614 = Multiply(x=w1561, y=10.0) -> (x*y=w1564:dbl)
                  n615 = Quotient & Remainder(x=w1564, y=2.0) -> (x-y*floor(x/y)=w1565:dbl)  [unwired: 1 out]
                  n616 = Subtract(x=w1564, y=w1565) -> (x-y=w1563:dbl)
                  n617 = Divide(x=w1563, y=10.0) -> (x/y=w1560:dbl)
                }
                frame "N" {
                  n618 = Multiply(x=w1570, y=1.0) -> (x*y=w1573:dbl)
                  n619 = Quotient & Remainder(x=w1573, y=2.0) -> (x-y*floor(x/y)=w1574:dbl)  [unwired: 1 out]
                  n620 = Subtract(x=w1573, y=w1574) -> (x-y=w1572:dbl)
                  n621 = Divide(x=w1572, y=1.0) -> (x/y=w1569:dbl)
                }
                frame "g" {
                }
                frame "daN" {
                  n622 = Multiply(x=w1580, y=10.0) -> (x*y=w1584:dbl)
                  n623 = Quotient & Remainder(x=w1584, y=2.0) -> (x-y*floor(x/y)=w1585:dbl)  [unwired: 1 out]
                  n624 = Subtract(x=w1584, y=w1585) -> (x-y=w1583:dbl)
                  n625 = Divide(x=w1583, y=10.0) -> (x/y=w1581:dbl)
                }
                frame "cN" {
                }
                frame "KN" {
                }
                frame "lb" {
                  n626 = Multiply(x=w1593, y=10.0) -> (x*y=w1597:dbl)
                  n627 = Quotient & Remainder(x=w1597, y=5.0) -> (x-y*floor(x/y)=w1598:dbl)  [unwired: 1 out]
                  n628 = Subtract(x=w1597, y=w1598) -> (x-y=w1596:dbl)
                  n629 = Divide(x=w1596, y=10.0) -> (x/y=w1594:dbl)
                }
              }
            }
          }
        }
        frame 9 {
          n630 = case shown="0, Default" w1604 {
            tunnel: [w1610 w1686] -> w1603
            tunnel: [w1609 w1685] -> w1602
            tunnel: w1606 -> [w1608 w1684]
            tunnel: w1605 -> [w1607 w1683]
            frame 0, Default {
              n631 = case shown="\"daN\"" w1607 {
                tunnel: [w1612 w1627 w1642 w1650 w1664 w1666 w1669] -> w1610
                tunnel: [3 2 0 3 0 0 2] -> w1609
                tunnel: w1608 -> [w1616 w1631 w1643 w1654 w1664 w1666 w1673]
                frame "Kg", Default {
                  n632 = Multiply(x=w1616, y=200.0) -> (x*y=w1619:dbl)
                  n633 = Quotient & Remainder(x=w1619, y=5.0) -> (x-y*floor(x/y)=w1620:dbl)  [unwired: 1 out]
                  n634 = Subtract(x=w1619, y=w1620) -> (x-y=w1618:dbl)
                  n635 = Divide(x=w1618, y=200.0) -> (x/y=w1613:dbl)
                  n636 = Absolute Value(x=w1613) -> (abs(x)=w1611:dbl)
                  n637 = Greater?(x=w1611, y=0.05) -> (0:w1615:bool)
                  n638 = case shown="False" w1615 {
                    tunnel: w1613 -> [_ w1625]
                    tunnel: [0.0 w1625] -> w1612
                    frame False {
                    }
                    frame True {
                    }
                  }
                }
                frame "N" {
                  n639 = Multiply(x=w1631, y=20.0) -> (x*y=w1634:dbl)
                  n640 = Quotient & Remainder(x=w1634, y=5.0) -> (x-y*floor(x/y)=w1635:dbl)  [unwired: 1 out]
                  n641 = Subtract(x=w1634, y=w1635) -> (x-y=w1633:dbl)
                  n642 = Divide(x=w1633, y=20.0) -> (x/y=w1628:dbl)
                  n643 = Absolute Value(x=w1628) -> (abs(x)=w1626:dbl)
                  n644 = Greater?(x=w1626, y=0.5) -> (0:w1630:bool)
                  n645 = case shown="False" w1630 {
                    tunnel: w1628 -> [_ w1640]
                    tunnel: [0.0 w1640] -> w1627
                    frame False {
                    }
                    frame True {
                    }
                  }
                }
                frame "g" {
                  n646 = Absolute Value(x=w1643) -> (abs(x)=w1641:dbl)
                  n647 = Greater?(x=w1641, y=2.0) -> (0:w1645:bool)
                  n648 = case shown="False" w1645 {
                    tunnel: w1643 -> [_ w1648]
                    tunnel: [0.0 w1648] -> w1642
                    frame False {
                    }
                    frame True {
                    }
                  }
                }
                frame "daN" {
                  n649 = Multiply(x=w1654, y=200.0) -> (x*y=w1657:dbl)
                  n650 = Quotient & Remainder(x=w1657, y=5.0) -> (x-y*floor(x/y)=w1658:dbl)  [unwired: 1 out]
                  n651 = Subtract(x=w1657, y=w1658) -> (x-y=w1656:dbl)
                  n652 = Divide(x=w1656, y=200.0) -> (x/y=w1651:dbl)
                  n653 = Absolute Value(x=w1651) -> (abs(x)=w1649:dbl)
                  n654 = Greater?(x=w1649, y=0.05) -> (0:w1653:bool)
                  n655 = case shown="False" w1653 {
                    tunnel: w1651 -> [_ w1663]
                    tunnel: [0.0 w1663] -> w1650
                    frame False {
                    }
                    frame True {
                    }
                  }
                }
                frame "cN" {
                }
                frame "KN" {
                }
                frame "lb" {
                  n656 = Multiply(x=w1673, y=100.0) -> (x*y=w1676:dbl)
                  n657 = Quotient & Remainder(x=w1676, y=5.0) -> (x-y*floor(x/y)=w1677:dbl)  [unwired: 1 out]
                  n658 = Subtract(x=w1676, y=w1677) -> (x-y=w1675:dbl)
                  n659 = Divide(x=w1675, y=100.0) -> (x/y=w1670:dbl)
                  n660 = Absolute Value(x=w1670) -> (abs(x)=w1668:dbl)
                  n661 = Greater?(x=w1668, y=0.1) -> (0:w1672:bool)
                  n662 = case shown="False" w1672 {
                    tunnel: w1670 -> [_ w1682]
                    tunnel: [0.0 w1682] -> w1669
                    frame False {
                    }
                    frame True {
                    }
                  }
                }
              }
            }
            frame 1 {
              n663 = case shown="\"lb\"" w1683 {
                tunnel: [w1687 w1696 w1705 w1708 w1716 w1718 w1721] -> w1686
                tunnel: [1 0 0 1 0 0 1] -> w1685
                tunnel: w1684 -> [w1688 w1697 w1705 w1707 w1716 w1718 w1720]
                frame "Kg", Default {
                  n664 = Multiply(x=w1688, y=10.0) -> (x*y=w1691:dbl)
                  n665 = Quotient & Remainder(x=w1691, y=2.0) -> (x-y*floor(x/y)=w1692:dbl)  [unwired: 1 out]
                  n666 = Subtract(x=w1691, y=w1692) -> (x-y=w1690:dbl)
                  n667 = Divide(x=w1690, y=10.0) -> (x/y=w1687:dbl)
                }
                frame "N" {
                  n668 = Multiply(x=w1697, y=1.0) -> (x*y=w1700:dbl)
                  n669 = Quotient & Remainder(x=w1700, y=2.0) -> (x-y*floor(x/y)=w1701:dbl)  [unwired: 1 out]
                  n670 = Subtract(x=w1700, y=w1701) -> (x-y=w1699:dbl)
                  n671 = Divide(x=w1699, y=1.0) -> (x/y=w1696:dbl)
                }
                frame "g" {
                }
                frame "daN" {
                  n672 = Multiply(x=w1707, y=10.0) -> (x*y=w1711:dbl)
                  n673 = Quotient & Remainder(x=w1711, y=2.0) -> (x-y*floor(x/y)=w1712:dbl)  [unwired: 1 out]
                  n674 = Subtract(x=w1711, y=w1712) -> (x-y=w1710:dbl)
                  n675 = Divide(x=w1710, y=10.0) -> (x/y=w1708:dbl)
                }
                frame "cN" {
                }
                frame "KN" {
                }
                frame "lb" {
                  n676 = Multiply(x=w1720, y=10.0) -> (x*y=w1724:dbl)
                  n677 = Quotient & Remainder(x=w1724, y=5.0) -> (x-y*floor(x/y)=w1725:dbl)  [unwired: 1 out]
                  n678 = Subtract(x=w1724, y=w1725) -> (x-y=w1723:dbl)
                  n679 = Divide(x=w1723, y=10.0) -> (x/y=w1721:dbl)
                }
              }
            }
          }
        }
        frame 20 {
          n680 = case shown="1" w1731 {
            tunnel: [w1737 w1814] -> w1730
            tunnel: [w1736 w1813] -> w1729
            tunnel: w1733 -> [w1735 w1812]
            tunnel: w1732 -> [w1734 w1811]
            frame 0, Default {
              n681 = case shown="\"lb\"" w1734 {
                tunnel: [w1739 w1754 w1768 w1771 w1785 w1787 w1797] -> w1737
                tunnel: [2 2 0 2 0 4 1] -> w1736
                tunnel: w1735 -> [w1743 w1758 w1768 w1775 w1785 w1788 w1801]
                frame "Kg", Default {
                  n682 = Multiply(x=w1743, y=20.0) -> (x*y=w1746:dbl)
                  n683 = Quotient & Remainder(x=w1746, y=5.0) -> (x-y*floor(x/y)=w1747:dbl)  [unwired: 1 out]
                  n684 = Subtract(x=w1746, y=w1747) -> (x-y=w1745:dbl)
                  n685 = Divide(x=w1745, y=20.0) -> (x/y=w1740:dbl)
                  n686 = Absolute Value(x=w1740) -> (abs(x)=w1738:dbl)
                  n687 = Greater?(x=w1738, y=0.5) -> (0:w1742:bool)
                  n688 = case shown="False" w1742 {
                    tunnel: w1740 -> [_ w1752]
                    tunnel: [0.0 w1752] -> w1739
                    frame False {
                    }
                    frame True {
                    }
                  }
                }
                frame "N" {
                  n689 = Multiply(x=w1758, y=2.0) -> (x*y=w1761:dbl)
                  n690 = Quotient & Remainder(x=w1761, y=5.0) -> (x-y*floor(x/y)=w1762:dbl)  [unwired: 1 out]
                  n691 = Subtract(x=w1761, y=w1762) -> (x-y=w1760:dbl)
                  n692 = Divide(x=w1760, y=2.0) -> (x/y=w1755:dbl)
                  n693 = Absolute Value(x=w1755) -> (abs(x)=w1753:dbl)
                  n694 = Greater?(x=w1753, y=5.0) -> (0:w1757:bool)
                  n695 = case shown="False" w1757 {
                    tunnel: w1755 -> [_ w1767]
                    tunnel: [0.0 w1767] -> w1754
                    frame False {
                    }
                    frame True {
                    }
                  }
                }
                frame "g" {
                }
                frame "daN" {
                  n696 = Multiply(x=w1775, y=200.0) -> (x*y=w1778:dbl)
                  n697 = Quotient & Remainder(x=w1778, y=5.0) -> (x-y*floor(x/y)=w1779:dbl)  [unwired: 1 out]
                  n698 = Subtract(x=w1778, y=w1779) -> (x-y=w1777:dbl)
                  n699 = Divide(x=w1777, y=200.0) -> (x/y=w1772:dbl)
                  n700 = Absolute Value(x=w1772) -> (abs(x)=w1770:dbl)
                  n701 = Greater?(x=w1770, y=0.05) -> (0:w1774:bool)
                  n702 = case shown="False" w1774 {
                    tunnel: w1772 -> [_ w1784]
                    tunnel: [0.0 w1784] -> w1771
                    frame False {
                    }
                    frame True {
                    }
                  }
                }
                frame "cN" {
                }
                frame "KN" {
                  n703 = Multiply(x=w1788, y=200.0) -> (x*y=w1791:dbl)
                  n704 = Quotient & Remainder(x=w1791, y=5.0) -> (x-y*floor(x/y)=w1792:dbl)  [unwired: 1 out]
                  n705 = Subtract(x=w1791, y=w1792) -> (x-y=w1790:dbl)
                  n706 = Divide(x=w1790, y=200.0) -> (x/y=w1787:dbl)
                }
                frame "lb" {
                  n707 = Multiply(x=w1801, y=10.0) -> (x*y=w1804:dbl)
                  n708 = Quotient & Remainder(x=w1804, y=5.0) -> (x-y*floor(x/y)=w1805:dbl)  [unwired: 1 out]
                  n709 = Subtract(x=w1804, y=w1805) -> (x-y=w1803:dbl)
                  n710 = Divide(x=w1803, y=10.0) -> (x/y=w1798:dbl)
                  n711 = Absolute Value(x=w1798) -> (abs(x)=w1796:dbl)
                  n712 = Greater?(x=w1796, y=1.0) -> (0:w1800:bool)
                  n713 = case shown="False" w1800 {
                    tunnel: w1798 -> [_ w1810]
                    tunnel: [0.0 w1810] -> w1797
                    frame False {
                    }
                    frame True {
                    }
                  }
                }
              }
            }
            frame 1 {
              n714 = case shown="\"KN\"" w1811 {
                tunnel: [w1816 w1831 w1846 w1854 w1868 w1870 w1880] -> w1814
                tunnel: [2 2 0 2 0 4 2] -> w1813
                tunnel: w1812 -> [w1820 w1835 w1847 w1858 w1868 w1871 w1884]
                frame "Kg", Default {
                  n715 = Multiply(x=w1820, y=200.0) -> (x*y=w1823:dbl)
                  n716 = Quotient & Remainder(x=w1823, y=5.0) -> (x-y*floor(x/y)=w1824:dbl)  [unwired: 1 out]
                  n717 = Subtract(x=w1823, y=w1824) -> (x-y=w1822:dbl)
                  n718 = Divide(x=w1822, y=200.0) -> (x/y=w1817:dbl)
                  n719 = Absolute Value(x=w1817) -> (abs(x)=w1815:dbl)
                  n720 = Greater?(x=w1815, y=0.05) -> (0:w1819:bool)
                  n721 = case shown="False" w1819 {
                    tunnel: w1817 -> [_ w1829]
                    tunnel: [0.0 w1829] -> w1816
                    frame False {
                    }
                    frame True {
                    }
                  }
                }
                frame "N" {
                  n722 = Multiply(x=w1835, y=20.0) -> (x*y=w1838:dbl)
                  n723 = Quotient & Remainder(x=w1838, y=5.0) -> (x-y*floor(x/y)=w1839:dbl)  [unwired: 1 out]
                  n724 = Subtract(x=w1838, y=w1839) -> (x-y=w1837:dbl)
                  n725 = Divide(x=w1837, y=20.0) -> (x/y=w1832:dbl)
                  n726 = Absolute Value(x=w1832) -> (abs(x)=w1830:dbl)
                  n727 = Greater?(x=w1830, y=0.5) -> (0:w1834:bool)
                  n728 = case shown="False" w1834 {
                    tunnel: w1832 -> [_ w1844]
                    tunnel: [0.0 w1844] -> w1831
                    frame False {
                    }
                    frame True {
                    }
                  }
                }
                frame "g" {
                  n729 = Absolute Value(x=w1847) -> (abs(x)=w1845:dbl)
                  n730 = Greater?(x=w1845, y=2.0) -> (0:w1849:bool)
                  n731 = case shown="False" w1849 {
                    tunnel: w1847 -> [_ w1852]
                    tunnel: [0.0 w1852] -> w1846
                    frame False {
                    }
                    frame True {
                    }
                  }
                }
                frame "daN" {
                  n732 = Multiply(x=w1858, y=200.0) -> (x*y=w1861:dbl)
                  n733 = Quotient & Remainder(x=w1861, y=5.0) -> (x-y*floor(x/y)=w1862:dbl)  [unwired: 1 out]
                  n734 = Subtract(x=w1861, y=w1862) -> (x-y=w1860:dbl)
                  n735 = Divide(x=w1860, y=200.0) -> (x/y=w1855:dbl)
                  n736 = Absolute Value(x=w1855) -> (abs(x)=w1853:dbl)
                  n737 = Greater?(x=w1853, y=0.05) -> (0:w1857:bool)
                  n738 = case shown="False" w1857 {
                    tunnel: w1855 -> [_ w1867]
                    tunnel: [0.0 w1867] -> w1854
                    frame False {
                    }
                    frame True {
                    }
                  }
                }
                frame "cN" {
                }
                frame "KN" {
                  n739 = Multiply(x=w1871, y=200.0) -> (x*y=w1874:dbl)
                  n740 = Quotient & Remainder(x=w1874, y=5.0) -> (x-y*floor(x/y)=w1875:dbl)  [unwired: 1 out]
                  n741 = Subtract(x=w1874, y=w1875) -> (x-y=w1873:dbl)
                  n742 = Divide(x=w1873, y=200.0) -> (x/y=w1870:dbl)
                }
                frame "lb" {
                  n743 = Multiply(x=w1884, y=100.0) -> (x*y=w1887:dbl)
                  n744 = Quotient & Remainder(x=w1887, y=5.0) -> (x-y*floor(x/y)=w1888:dbl)  [unwired: 1 out]
                  n745 = Subtract(x=w1887, y=w1888) -> (x-y=w1886:dbl)
                  n746 = Divide(x=w1886, y=100.0) -> (x/y=w1881:dbl)
                  n747 = Absolute Value(x=w1881) -> (abs(x)=w1879:dbl)
                  n748 = Greater?(x=w1879, y=0.1) -> (0:w1883:bool)
                  n749 = case shown="False" w1883 {
                    tunnel: w1881 -> [_ w1893]
                    tunnel: [0.0 w1893] -> w1880
                    frame False {
                    }
                    frame True {
                    }
                  }
                }
              }
            }
          }
        }
        frame 19 {
          n750 = case shown="0, Default" w1896 {
            tunnel: [w1902 w1991] -> w1895
            tunnel: [w1901 w1990] -> w1894
            tunnel: w1898 -> [w1900 w1989]
            tunnel: w1897 -> [w1899 w1988]
            frame 0, Default {
              n751 = case shown="\"KN\"" w1899 {
                tunnel: [w1904 w1919 w1934 w1942 w1956 w1958 w1974] -> w1902
                tunnel: [3 2 0 3 0 0 2] -> w1901
                tunnel: w1900 -> [w1908 w1923 w1935 w1946 w1956 w1963 w1978]
                frame "Kg", Default {
                  n752 = Multiply(x=w1908, y=200.0) -> (x*y=w1911:dbl)
                  n753 = Quotient & Remainder(x=w1911, y=5.0) -> (x-y*floor(x/y)=w1912:dbl)  [unwired: 1 out]
                  n754 = Subtract(x=w1911, y=w1912) -> (x-y=w1910:dbl)
                  n755 = Divide(x=w1910, y=200.0) -> (x/y=w1905:dbl)
                  n756 = Absolute Value(x=w1905) -> (abs(x)=w1903:dbl)
                  n757 = Greater?(x=w1903, y=0.05) -> (0:w1907:bool)
                  n758 = case shown="False" w1907 {
                    tunnel: w1905 -> [_ w1917]
                    tunnel: [0.0 w1917] -> w1904
                    frame False {
                    }
                    frame True {
                    }
                  }
                }
                frame "N" {
                  n759 = Multiply(x=w1923, y=20.0) -> (x*y=w1926:dbl)
                  n760 = Quotient & Remainder(x=w1926, y=5.0) -> (x-y*floor(x/y)=w1927:dbl)  [unwired: 1 out]
                  n761 = Subtract(x=w1926, y=w1927) -> (x-y=w1925:dbl)
                  n762 = Divide(x=w1925, y=20.0) -> (x/y=w1920:dbl)
                  n763 = Absolute Value(x=w1920) -> (abs(x)=w1918:dbl)
                  n764 = Greater?(x=w1918, y=0.5) -> (0:w1922:bool)
                  n765 = case shown="False" w1922 {
                    tunnel: w1920 -> [_ w1932]
                    tunnel: [0.0 w1932] -> w1919
                    frame False {
                    }
                    frame True {
                    }
                  }
                }
                frame "g" {
                  n766 = Absolute Value(x=w1935) -> (abs(x)=w1933:dbl)
                  n767 = Greater?(x=w1933, y=2.0) -> (0:w1937:bool)
                  n768 = case shown="False" w1937 {
                    tunnel: w1935 -> [_ w1940]
                    tunnel: [0.0 w1940] -> w1934
                    frame False {
                    }
                    frame True {
                    }
                  }
                }
                frame "daN" {
                  n769 = Multiply(x=w1946, y=200.0) -> (x*y=w1949:dbl)
                  n770 = Quotient & Remainder(x=w1949, y=5.0) -> (x-y*floor(x/y)=w1950:dbl)  [unwired: 1 out]
                  n771 = Subtract(x=w1949, y=w1950) -> (x-y=w1948:dbl)
                  n772 = Divide(x=w1948, y=200.0) -> (x/y=w1943:dbl)
                  n773 = Absolute Value(x=w1943) -> (abs(x)=w1941:dbl)
                  n774 = Greater?(x=w1941, y=0.05) -> (0:w1945:bool)
                  n775 = case shown="False" w1945 {
                    tunnel: w1943 -> [_ w1955]
                    tunnel: [0.0 w1955] -> w1942
                    frame False {
                    }
                    frame True {
                    }
                  }
                }
                frame "cN" {
                }
                frame "KN" {
                  n776 = Multiply(x=w1963, y=2000.0) -> (x*y=w1966:dbl)
                  n777 = Quotient & Remainder(x=w1966, y=5.0) -> (x-y*floor(x/y)=w1967:dbl)  [unwired: 1 out]
                  n778 = Subtract(x=w1966, y=w1967) -> (x-y=w1965:dbl)
                  n779 = Divide(x=w1965, y=2000.0) -> (x/y=w1959:dbl)
                  n780 = Absolute Value(x=w1959) -> (abs(x)=w1960:dbl)
                  n781 = Greater?(x=w1960, y=0.0005) -> (0:w1962:bool)
                  n782 = case shown="False" w1962 {
                    tunnel: w1959 -> [_ w1972]
                    tunnel: [0.0 w1972] -> w1958
                    frame False {
                    }
                    frame True {
                    }
                  }
                }
                frame "lb" {
                  n783 = Multiply(x=w1978, y=100.0) -> (x*y=w1981:dbl)
                  n784 = Quotient & Remainder(x=w1981, y=5.0) -> (x-y*floor(x/y)=w1982:dbl)  [unwired: 1 out]
                  n785 = Subtract(x=w1981, y=w1982) -> (x-y=w1980:dbl)
                  n786 = Divide(x=w1980, y=100.0) -> (x/y=w1975:dbl)
                  n787 = Absolute Value(x=w1975) -> (abs(x)=w1973:dbl)
                  n788 = Greater?(x=w1973, y=0.1) -> (0:w1977:bool)
                  n789 = case shown="False" w1977 {
                    tunnel: w1975 -> [_ w1987]
                    tunnel: [0.0 w1987] -> w1974
                    frame False {
                    }
                    frame True {
                    }
                  }
                }
              }
            }
            frame 1 {
              n790 = case shown="\"KN\"" w1988 {
                tunnel: [w1993 w2008 w2023 w2031 w2045 w2047 w2057] -> w1991
                tunnel: [3 2 0 3 0 0 2] -> w1990
                tunnel: w1989 -> [w1997 w2012 w2024 w2035 w2045 w2048 w2061]
                frame "Kg", Default {
                  n791 = Multiply(x=w1997, y=200.0) -> (x*y=w2000:dbl)
                  n792 = Quotient & Remainder(x=w2000, y=5.0) -> (x-y*floor(x/y)=w2001:dbl)  [unwired: 1 out]
                  n793 = Subtract(x=w2000, y=w2001) -> (x-y=w1999:dbl)
                  n794 = Divide(x=w1999, y=200.0) -> (x/y=w1994:dbl)
                  n795 = Absolute Value(x=w1994) -> (abs(x)=w1992:dbl)
                  n796 = Greater?(x=w1992, y=0.05) -> (0:w1996:bool)
                  n797 = case shown="False" w1996 {
                    tunnel: w1994 -> [_ w2006]
                    tunnel: [0.0 w2006] -> w1993
                    frame False {
                    }
                    frame True {
                    }
                  }
                }
                frame "N" {
                  n798 = Multiply(x=w2012, y=20.0) -> (x*y=w2015:dbl)
                  n799 = Quotient & Remainder(x=w2015, y=5.0) -> (x-y*floor(x/y)=w2016:dbl)  [unwired: 1 out]
                  n800 = Subtract(x=w2015, y=w2016) -> (x-y=w2014:dbl)
                  n801 = Divide(x=w2014, y=20.0) -> (x/y=w2009:dbl)
                  n802 = Absolute Value(x=w2009) -> (abs(x)=w2007:dbl)
                  n803 = Greater?(x=w2007, y=0.5) -> (0:w2011:bool)
                  n804 = case shown="False" w2011 {
                    tunnel: w2009 -> [_ w2021]
                    tunnel: [0.0 w2021] -> w2008
                    frame False {
                    }
                    frame True {
                    }
                  }
                }
                frame "g" {
                  n805 = Absolute Value(x=w2024) -> (abs(x)=w2022:dbl)
                  n806 = Greater?(x=w2022, y=2.0) -> (0:w2026:bool)
                  n807 = case shown="False" w2026 {
                    tunnel: w2024 -> [_ w2029]
                    tunnel: [0.0 w2029] -> w2023
                    frame False {
                    }
                    frame True {
                    }
                  }
                }
                frame "daN" {
                  n808 = Multiply(x=w2035, y=200.0) -> (x*y=w2038:dbl)
                  n809 = Quotient & Remainder(x=w2038, y=5.0) -> (x-y*floor(x/y)=w2039:dbl)  [unwired: 1 out]
                  n810 = Subtract(x=w2038, y=w2039) -> (x-y=w2037:dbl)
                  n811 = Divide(x=w2037, y=200.0) -> (x/y=w2032:dbl)
                  n812 = Absolute Value(x=w2032) -> (abs(x)=w2030:dbl)
                  n813 = Greater?(x=w2030, y=0.05) -> (0:w2034:bool)
                  n814 = case shown="False" w2034 {
                    tunnel: w2032 -> [_ w2044]
                    tunnel: [0.0 w2044] -> w2031
                    frame False {
                    }
                    frame True {
                    }
                  }
                }
                frame "cN" {
                }
                frame "KN" {
                  n815 = Multiply(x=w2048, y=2000.0) -> (x*y=w2051:dbl)
                  n816 = Quotient & Remainder(x=w2051, y=5.0) -> (x-y*floor(x/y)=w2052:dbl)  [unwired: 1 out]
                  n817 = Subtract(x=w2051, y=w2052) -> (x-y=w2050:dbl)
                  n818 = Divide(x=w2050, y=2000.0) -> (x/y=w2047:dbl)
                }
                frame "lb" {
                  n819 = Multiply(x=w2061, y=100.0) -> (x*y=w2064:dbl)
                  n820 = Quotient & Remainder(x=w2064, y=5.0) -> (x-y*floor(x/y)=w2065:dbl)  [unwired: 1 out]
                  n821 = Subtract(x=w2064, y=w2065) -> (x-y=w2063:dbl)
                  n822 = Divide(x=w2063, y=100.0) -> (x/y=w2058:dbl)
                  n823 = Absolute Value(x=w2058) -> (abs(x)=w2056:dbl)
                  n824 = Greater?(x=w2056, y=0.1) -> (0:w2060:bool)
                  n825 = case shown="False" w2060 {
                    tunnel: w2058 -> [_ w2070]
                    tunnel: [0.0 w2070] -> w2057
                    frame False {
                    }
                    frame True {
                    }
                  }
                }
              }
            }
          }
        }
        frame 10 {
          n826 = case shown="0, Default" w2073 {
            tunnel: w2074 -> [w2079 w2155]
            tunnel: [w2078 w2154] -> w2071
            tunnel: [w2077 w2153] -> w2072
            tunnel: w2075 -> [w2076 w2152]
            frame 0, Default {
              n827 = case shown="\"lb\"" w2079 {
                tunnel: [w2081 w2096 w2110 w2113 w2127 w2131 w2145] -> w2078
                tunnel: [2 1 0 2 0 4 1] -> w2077
                tunnel: w2076 -> [w2085 w2100 w2110 w2117 w2127 w2134 w2146]
                frame "Kg", Default {
                  n828 = Multiply(x=w2085, y=100.0) -> (x*y=w2088:dbl)
                  n829 = Quotient & Remainder(x=w2088, y=5.0) -> (x-y*floor(x/y)=w2089:dbl)  [unwired: 1 out]
                  n830 = Subtract(x=w2088, y=w2089) -> (x-y=w2087:dbl)
                  n831 = Divide(x=w2087, y=100.0) -> (x/y=w2082:dbl)
                  n832 = Absolute Value(x=w2082) -> (abs(x)=w2080:dbl)
                  n833 = Greater?(x=w2080, y=0.1) -> (0:w2084:bool)
                  n834 = case shown="False" w2084 {
                    tunnel: w2082 -> [_ w2094]
                    tunnel: [0.0 w2094] -> w2081
                    frame False {
                    }
                    frame True {
                    }
                  }
                }
                frame "N" {
                  n835 = Multiply(x=w2100, y=10.0) -> (x*y=w2103:dbl)
                  n836 = Quotient & Remainder(x=w2103, y=5.0) -> (x-y*floor(x/y)=w2104:dbl)  [unwired: 1 out]
                  n837 = Subtract(x=w2103, y=w2104) -> (x-y=w2102:dbl)
                  n838 = Divide(x=w2102, y=10.0) -> (x/y=w2097:dbl)
                  n839 = Absolute Value(x=w2097) -> (abs(x)=w2095:dbl)
                  n840 = Greater?(x=w2095, y=1.0) -> (0:w2099:bool)
                  n841 = case shown="False" w2099 {
                    tunnel: w2097 -> [_ w2109]
                    tunnel: [0.0 w2109] -> w2096
                    frame False {
                    }
                    frame True {
                    }
                  }
                }
                frame "g" {
                }
                frame "daN" {
                  n842 = Multiply(x=w2117, y=100.0) -> (x*y=w2120:dbl)
                  n843 = Quotient & Remainder(x=w2120, y=5.0) -> (x-y*floor(x/y)=w2121:dbl)  [unwired: 1 out]
                  n844 = Subtract(x=w2120, y=w2121) -> (x-y=w2119:dbl)
                  n845 = Divide(x=w2119, y=100.0) -> (x/y=w2114:dbl)
                  n846 = Absolute Value(x=w2114) -> (abs(x)=w2112:dbl)
                  n847 = Greater?(x=w2112, y=0.1) -> (0:w2116:bool)
                  n848 = case shown="False" w2116 {
                    tunnel: w2114 -> [_ w2126]
                    tunnel: [0.0 w2126] -> w2113
                    frame False {
                    }
                    frame True {
                    }
                  }
                }
                frame "cN" {
                }
                frame "KN" {
                  n849 = Multiply(x=w2134, y=10000.0) -> (x*y=w2137:dbl)
                  n850 = Quotient & Remainder(x=w2137, y=5.0) -> (x-y*floor(x/y)=w2138:dbl)  [unwired: 1 out]
                  n851 = Subtract(x=w2137, y=w2138) -> (x-y=w2136:dbl)
                  n852 = Divide(x=w2136, y=10000.0) -> (x/y=w2130:dbl)
                  n853 = Absolute Value(x=w2130) -> (abs(x)=w2129:dbl)
                  n854 = Greater?(x=w2129, y=0.001) -> (0:w2133:bool)
                  n855 = case shown="False" w2133 {
                    tunnel: w2130 -> [_ w2143]
                    tunnel: [0.0 w2143] -> w2131
                    frame False {
                    }
                    frame True {
                    }
                  }
                }
                frame "lb" {
                  n856 = Absolute Value(x=w2146) -> (abs(x)=w2144:dbl)
                  n857 = Greater?(x=w2144, y=0.2) -> (0:w2148:bool)
                  n858 = case shown="False" w2148 {
                    tunnel: w2146 -> [_ w2151]
                    tunnel: [0.0 w2151] -> w2145
                    frame False {
                    }
                    frame True {
                    }
                  }
                }
              }
            }
            frame 1 {
              n859 = case shown="\"KN\"" w2155 {
                tunnel: [w2157 w2166 w2175 w2184 w2192 w2194 w2204] -> w2154
                tunnel: [2 1 0 2 0 4 1] -> w2153
                tunnel: w2152 -> [w2156 w2165 w2174 w2183 w2192 w2195 w2203]
                frame "Kg", Default {
                  n860 = Multiply(x=w2156, y=20.0) -> (x*y=w2160:dbl)
                  n861 = Quotient & Remainder(x=w2160, y=5.0) -> (x-y*floor(x/y)=w2161:dbl)  [unwired: 1 out]
                  n862 = Subtract(x=w2160, y=w2161) -> (x-y=w2159:dbl)
                  n863 = Divide(x=w2159, y=20.0) -> (x/y=w2157:dbl)
                }
                frame "N" {
                  n864 = Multiply(x=w2165, y=2.0) -> (x*y=w2169:dbl)
                  n865 = Quotient & Remainder(x=w2169, y=5.0) -> (x-y*floor(x/y)=w2170:dbl)  [unwired: 1 out]
                  n866 = Subtract(x=w2169, y=w2170) -> (x-y=w2168:dbl)
                  n867 = Divide(x=w2168, y=2.0) -> (x/y=w2166:dbl)
                }
                frame "g" {
                  n868 = Multiply(x=w2174, y=20.0) -> (x*y=w2178:dbl)
                  n869 = Quotient & Remainder(x=w2178, y=5.0) -> (x-y*floor(x/y)=w2179:dbl)  [unwired: 1 out]
                  n870 = Subtract(x=w2178, y=w2179) -> (x-y=w2177:dbl)
                  n871 = Divide(x=w2177, y=20.0) -> (x/y=w2175:dbl)
                }
                frame "daN" {
                  n872 = Multiply(x=w2183, y=20.0) -> (x*y=w2187:dbl)
                  n873 = Quotient & Remainder(x=w2187, y=5.0) -> (x-y*floor(x/y)=w2188:dbl)  [unwired: 1 out]
                  n874 = Subtract(x=w2187, y=w2188) -> (x-y=w2186:dbl)
                  n875 = Divide(x=w2186, y=20.0) -> (x/y=w2184:dbl)
                }
                frame "cN" {
                }
                frame "KN" {
                  n876 = Multiply(x=w2195, y=2000.0) -> (x*y=w2198:dbl)
                  n877 = Quotient & Remainder(x=w2198, y=5.0) -> (x-y*floor(x/y)=w2199:dbl)  [unwired: 1 out]
                  n878 = Subtract(x=w2198, y=w2199) -> (x-y=w2197:dbl)
                  n879 = Divide(x=w2197, y=2000.0) -> (x/y=w2194:dbl)
                }
                frame "lb" {
                  n880 = Multiply(x=w2203, y=10.0) -> (x*y=w2207:dbl)
                  n881 = Quotient & Remainder(x=w2207, y=5.0) -> (x-y*floor(x/y)=w2208:dbl)  [unwired: 1 out]
                  n882 = Subtract(x=w2207, y=w2208) -> (x-y=w2206:dbl)
                  n883 = Divide(x=w2206, y=10.0) -> (x/y=w2204:dbl)
                }
              }
            }
          }
        }
        frame 11 {
          n884 = case shown="0, Default" w2214 {
            tunnel: [w2220 w2275] -> w2213
            tunnel: [w2219 w2274] -> w2212
            tunnel: w2216 -> [w2218 w2273]
            tunnel: w2215 -> [w2217 w2272]
            frame 0, Default {
              n885 = case shown="\"KN\"" w2217 {
                tunnel: [w2222 w2230 w2237 w2240 w2247 w2250 w2258] -> w2220
                tunnel: [1 0 0 1 0 3 1] -> w2219
                tunnel: w2218 -> [w2223 w2231 w2237 w2241 w2247 w2251 w2262]
                frame "Kg", Default {
                  n886 = Absolute Value(x=w2223) -> (abs(x)=w2221:dbl)
                  n887 = Greater?(x=w2221, y=0.2) -> (0:w2225:bool)
                  n888 = case shown="False" w2225 {
                    tunnel: w2223 -> [_ w2228]
                    tunnel: [0.0 w2228] -> w2222
                    frame False {
                    }
                    frame True {
                    }
                  }
                }
                frame "N" {
                  n889 = Absolute Value(x=w2231) -> (abs(x)=w2229:dbl)
                  n890 = Greater?(x=w2229, y=2.0) -> (0:w2233:bool)
                  n891 = case shown="False" w2233 {
                    tunnel: w2231 -> [_ w2236]
                    tunnel: [0.0 w2236] -> w2230
                    frame False {
                    }
                    frame True {
                    }
                  }
                }
                frame "g" {
                }
                frame "daN" {
                  n892 = Absolute Value(x=w2241) -> (abs(x)=w2239:dbl)
                  n893 = Greater?(x=w2239, y=0.2) -> (0:w2243:bool)
                  n894 = case shown="False" w2243 {
                    tunnel: w2241 -> [_ w2246]
                    tunnel: [0.0 w2246] -> w2240
                    frame False {
                    }
                    frame True {
                    }
                  }
                }
                frame "cN" {
                }
                frame "KN" {
                  n895 = Absolute Value(x=w2251) -> (abs(x)=w2249:dbl)
                  n896 = Greater?(x=w2249, y=0.002) -> (0:w2253:bool)
                  n897 = case shown="True" w2253 {
                    tunnel: w2251 -> [_ w2256]
                    tunnel: [0.0 w2256] -> w2250
                    frame False {
                    }
                    frame True {
                    }
                  }
                }
                frame "lb" {
                  n898 = Multiply(x=w2262, y=10.0) -> (x*y=w2265:dbl)
                  n899 = Quotient & Remainder(x=w2265, y=2.0) -> (x-y*floor(x/y)=w2266:dbl)  [unwired: 1 out]
                  n900 = Subtract(x=w2265, y=w2266) -> (x-y=w2264:dbl)
                  n901 = Divide(x=w2264, y=10.0) -> (x/y=w2259:dbl)
                  n902 = Absolute Value(x=w2259) -> (abs(x)=w2257:dbl)
                  n903 = Greater?(x=w2257, y=0.4) -> (0:w2261:bool)
                  n904 = case shown="False" w2261 {
                    tunnel: w2259 -> [_ w2271]
                    tunnel: [0.0 w2271] -> w2258
                    frame False {
                    }
                    frame True {
                    }
                  }
                }
              }
            }
            frame 1 {
              n905 = case shown="\"Kg\", Default" w2272 {
                tunnel: [w2277 w2285 w2294 w2296 w2305 w2307 w2309] -> w2275
                tunnel: [1 0 0 1 0 0 3] -> w2274
                tunnel: w2273 -> [w2276 w2286 w2294 w2297 w2305 w2307 w2310]
                frame "Kg", Default {
                  n906 = Multiply(x=w2276, y=10.0) -> (x*y=w2280:dbl)
                  n907 = Quotient & Remainder(x=w2280, y=5.0) -> (x-y*floor(x/y)=w2281:dbl)  [unwired: 1 out]
                  n908 = Subtract(x=w2280, y=w2281) -> (x-y=w2279:dbl)
                  n909 = Divide(x=w2279, y=10.0) -> (x/y=w2277:dbl)
                }
                frame "N" {
                  n910 = Multiply(x=w2286, y=1.0) -> (x*y=w2289:dbl)
                  n911 = Quotient & Remainder(x=w2289, y=5.0) -> (x-y*floor(x/y)=w2290:dbl)  [unwired: 1 out]
                  n912 = Subtract(x=w2289, y=w2290) -> (x-y=w2288:dbl)
                  n913 = Divide(x=w2288, y=1.0) -> (x/y=w2285:dbl)
                }
                frame "g" {
                }
                frame "daN" {
                  n914 = Multiply(x=w2297, y=10.0) -> (x*y=w2300:dbl)
                  n915 = Quotient & Remainder(x=w2300, y=5.0) -> (x-y*floor(x/y)=w2301:dbl)  [unwired: 1 out]
                  n916 = Subtract(x=w2300, y=w2301) -> (x-y=w2299:dbl)
                  n917 = Divide(x=w2299, y=10.0) -> (x/y=w2296:dbl)
                }
                frame "cN" {
                }
                frame "KN" {
                }
                frame "lb" {
                  n918 = Multiply(x=w2310, y=1000.0) -> (x*y=w2313:dbl)
                  n919 = Quotient & Remainder(x=w2313, y=5.0) -> (x-y*floor(x/y)=w2314:dbl)  [unwired: 1 out]
                  n920 = Subtract(x=w2313, y=w2314) -> (x-y=w2312:dbl)
                  n921 = Divide(x=w2312, y=1000.0) -> (x/y=w2309:dbl)
                }
              }
            }
          }
        }
        frame 12 {
          n922 = case shown="0, Default" w2320 {
            tunnel: [w2326 w2409] -> w2318
            tunnel: [w2325 w2408] -> w2319
            tunnel: w2322 -> [w2324 w2407]
            tunnel: w2321 -> [w2323 w2406]
            frame 0, Default {
              n923 = case shown="\"cN\"" w2323 {
                tunnel: [w2328 w2343 w2357 w2360 w2374 w2377 w2392] -> w2326
                tunnel: [1 0 0 1 0 3 1] -> w2325
                tunnel: w2324 -> [w2332 w2347 w2357 w2364 w2374 w2381 w2396]
                frame "Kg", Default {
                  n924 = Multiply(x=w2332, y=10.0) -> (x*y=w2335:dbl)
                  n925 = Quotient & Remainder(x=w2335, y=2.0) -> (x-y*floor(x/y)=w2336:dbl)  [unwired: 1 out]
                  n926 = Subtract(x=w2335, y=w2336) -> (x-y=w2334:dbl)
                  n927 = Divide(x=w2334, y=10.0) -> (x/y=w2329:dbl)
                  n928 = Absolute Value(x=w2329) -> (abs(x)=w2327:dbl)
                  n929 = Greater?(x=w2327, y=0.4) -> (0:w2331:bool)
                  n930 = case shown="False" w2331 {
                    tunnel: w2329 -> [_ w2341]
                    tunnel: [0.0 w2341] -> w2328
                    frame False {
                    }
                    frame True {
                    }
                  }
                }
                frame "N" {
                  n931 = Multiply(x=w2347, y=1.0) -> (x*y=w2350:dbl)
                  n932 = Quotient & Remainder(x=w2350, y=2.0) -> (x-y*floor(x/y)=w2351:dbl)  [unwired: 1 out]
                  n933 = Subtract(x=w2350, y=w2351) -> (x-y=w2349:dbl)
                  n934 = Divide(x=w2349, y=1.0) -> (x/y=w2344:dbl)
                  n935 = Absolute Value(x=w2344) -> (abs(x)=w2342:dbl)
                  n936 = Greater?(x=w2342, y=4.0) -> (0:w2346:bool)
                  n937 = case shown="False" w2346 {
                    tunnel: w2344 -> [_ w2356]
                    tunnel: [0.0 w2356] -> w2343
                    frame False {
                    }
                    frame True {
                    }
                  }
                }
                frame "g" {
                }
                frame "daN" {
                  n938 = Multiply(x=w2364, y=10.0) -> (x*y=w2367:dbl)
                  n939 = Quotient & Remainder(x=w2367, y=2.0) -> (x-y*floor(x/y)=w2368:dbl)  [unwired: 1 out]
                  n940 = Subtract(x=w2367, y=w2368) -> (x-y=w2366:dbl)
                  n941 = Divide(x=w2366, y=10.0) -> (x/y=w2361:dbl)
                  n942 = Absolute Value(x=w2361) -> (abs(x)=w2359:dbl)
                  n943 = Greater?(x=w2359, y=0.4) -> (0:w2363:bool)
                  n944 = case shown="False" w2363 {
                    tunnel: w2361 -> [_ w2373]
                    tunnel: [0.0 w2373] -> w2360
                    frame False {
                    }
                    frame True {
                    }
                  }
                }
                frame "cN" {
                }
                frame "KN" {
                  n945 = Multiply(x=w2381, y=1000.0) -> (x*y=w2384:dbl)
                  n946 = Quotient & Remainder(x=w2384, y=2.0) -> (x-y*floor(x/y)=w2385:dbl)  [unwired: 1 out]
                  n947 = Subtract(x=w2384, y=w2385) -> (x-y=w2383:dbl)
                  n948 = Divide(x=w2383, y=1000.0) -> (x/y=w2378:dbl)
                  n949 = Absolute Value(x=w2378) -> (abs(x)=w2376:dbl)
                  n950 = Greater?(x=w2376, y=0.004) -> (0:w2380:bool)
                  n951 = case shown="False" w2380 {
                    tunnel: w2378 -> [_ w2390]
                    tunnel: [0.0 w2390] -> w2377
                    frame False {
                    }
                    frame True {
                    }
                  }
                }
                frame "lb" {
                  n952 = Multiply(x=w2396, y=10.0) -> (x*y=w2399:dbl)
                  n953 = Quotient & Remainder(x=w2399, y=5.0) -> (x-y*floor(x/y)=w2400:dbl)  [unwired: 1 out]
                  n954 = Subtract(x=w2399, y=w2400) -> (x-y=w2398:dbl)
                  n955 = Divide(x=w2398, y=10.0) -> (x/y=w2393:dbl)
                  n956 = Absolute Value(x=w2393) -> (abs(x)=w2391:dbl)
                  n957 = Greater?(x=w2391, y=1.0) -> (0:w2395:bool)
                  n958 = case shown="False" w2395 {
                    tunnel: w2393 -> [_ w2405]
                    tunnel: [0.0 w2405] -> w2392
                    frame False {
                    }
                    frame True {
                    }
                  }
                }
              }
            }
            frame 1 {
              n959 = case shown="\"lb\"" w2406 {
                tunnel: [w2410 w2414 w2418 w2420 w2422 w2425 w2433] -> w2409
                tunnel: [0 0 0 0 0 2 1] -> w2408
                tunnel: w2407 -> [w2410 w2415 w2418 w2420 w2422 w2424 w2432]
                frame "Kg", Default {
                }
                frame "N" {
                  w2416 = 10.0 ("y")
                  n960 = Divide(x=w2415, y=w2416) -> (x/y=w2413:dbl)
                  n961 = To Word Integer(number=w2413) -> (16bit integer=w2412:i16)
                  n962 = Multiply(x=w2412, y=w2416) -> (x*y=w2414:dbl)
                }
                frame "g" {
                }
                frame "daN" {
                }
                frame "cN" {
                }
                frame "KN" {
                  n963 = Absolute Value(x=w2424) -> (abs(x)=w2426:dbl)
                  n964 = Greater?(x=w2426, y=0.02) -> (0:w2428:bool)
                  n965 = case shown="False" w2428 {
                    tunnel: w2424 -> [_ w2431]
                    tunnel: [0.0 w2431] -> w2425
                    frame False {
                    }
                    frame True {
                    }
                  }
                }
                frame "lb" {
                  n966 = Multiply(x=w2432, y=2.0) -> (x*y=w2436:dbl)
                  n967 = Quotient & Remainder(x=w2436, y=5.0) -> (x-y*floor(x/y)=w2437:dbl)  [unwired: 1 out]
                  n968 = Subtract(x=w2436, y=w2437) -> (x-y=w2435:dbl)
                  n969 = Divide(x=w2435, y=2.0) -> (x/y=w2433:dbl)
                }
              }
            }
          }
        }
        frame 13 {
          n970 = case shown="1" w2443 {
            tunnel: [w2449 w2512] -> w2442
            tunnel: [w2448 w2511] -> w2441
            tunnel: w2445 -> [w2447 w2510]
            tunnel: w2444 -> [w2446 w2509]
            frame 0, Default {
              n971 = case shown="\"KN\"" w2446 {
                tunnel: [w2451 w2465 w2467 w2470 w2484 w2488 w2502] -> w2449
                tunnel: [1 0 0 1 0 3 0] -> w2448
                tunnel: w2447 -> [w2455 w2465 w2467 w2474 w2484 w2491 w2503]
                frame "Kg", Default {
                  n972 = Multiply(x=w2455, y=10.0) -> (x*y=w2458:dbl)
                  n973 = Quotient & Remainder(x=w2458, y=5.0) -> (x-y*floor(x/y)=w2459:dbl)  [unwired: 1 out]
                  n974 = Subtract(x=w2458, y=w2459) -> (x-y=w2457:dbl)
                  n975 = Divide(x=w2457, y=10.0) -> (x/y=w2452:dbl)
                  n976 = Absolute Value(x=w2452) -> (abs(x)=w2450:dbl)
                  n977 = Greater?(x=w2450, y=1.0) -> (0:w2454:bool)
                  n978 = case shown="False" w2454 {
                    tunnel: w2452 -> [_ w2464]
                    tunnel: [0.0 w2464] -> w2451
                    frame False {
                    }
                    frame True {
                    }
                  }
                }
                frame "N" {
                }
                frame "g" {
                }
                frame "daN" {
                  n979 = Multiply(x=w2474, y=10.0) -> (x*y=w2477:dbl)
                  n980 = Quotient & Remainder(x=w2477, y=5.0) -> (x-y*floor(x/y)=w2478:dbl)  [unwired: 1 out]
                  n981 = Subtract(x=w2477, y=w2478) -> (x-y=w2476:dbl)
                  n982 = Divide(x=w2476, y=10.0) -> (x/y=w2471:dbl)
                  n983 = Absolute Value(x=w2471) -> (abs(x)=w2469:dbl)
                  n984 = Greater?(x=w2469, y=1.0) -> (0:w2473:bool)
                  n985 = case shown="False" w2473 {
                    tunnel: w2471 -> [_ w2483]
                    tunnel: [0.0 w2483] -> w2470
                    frame False {
                    }
                    frame True {
                    }
                  }
                }
                frame "cN" {
                }
                frame "KN" {
                  n986 = Multiply(x=w2491, y=1000.0) -> (x*y=w2494:dbl)
                  n987 = Quotient & Remainder(x=w2494, y=5.0) -> (x-y*floor(x/y)=w2495:dbl)  [unwired: 1 out]
                  n988 = Subtract(x=w2494, y=w2495) -> (x-y=w2493:dbl)
                  n989 = Divide(x=w2493, y=1000.0) -> (x/y=w2486:dbl)
                  n990 = Absolute Value(x=w2486) -> (abs(x)=w2487:dbl)
                  n991 = Greater?(x=w2487, y=0.01) -> (0:w2490:bool)
                  n992 = case shown="False" w2490 {
                    tunnel: w2486 -> [_ w2500]
                    tunnel: [0.0 w2500] -> w2488
                    frame False {
                    }
                    frame True {
                    }
                  }
                }
                frame "lb" {
                  n993 = Absolute Value(x=w2503) -> (abs(x)=w2501:dbl)
                  n994 = Greater?(x=w2501, y=2.0) -> (0:w2505:bool)
                  n995 = case shown="False" w2505 {
                    tunnel: w2503 -> [_ w2508]
                    tunnel: [0.0 w2508] -> w2502
                    frame False {
                    }
                    frame True {
                    }
                  }
                }
              }
            }
            frame 1 {
              n996 = case shown="\"N\"" w2509 {
                tunnel: [w2514 w2523 w2532 w2541 w2549 w2551 w2561] -> w2512
                tunnel: [2 1 0 2 0 4 1] -> w2511
                tunnel: w2510 -> [w2513 w2522 w2531 w2540 w2549 w2552 w2560]
                frame "Kg", Default {
                  n997 = Multiply(x=w2513, y=2.0) -> (x*y=w2517:dbl)
                  n998 = Quotient & Remainder(x=w2517, y=5.0) -> (x-y*floor(x/y)=w2518:dbl)  [unwired: 1 out]
                  n999 = Subtract(x=w2517, y=w2518) -> (x-y=w2516:dbl)
                  n1000 = Divide(x=w2516, y=2.0) -> (x/y=w2514:dbl)
                }
                frame "N" {
                  n1001 = Multiply(x=w2522, y=2.0) -> (x*y=w2526:dbl)
                  n1002 = Quotient & Remainder(x=w2526, y=5.0) -> (x-y*floor(x/y)=w2527:dbl)  [unwired: 1 out]
                  n1003 = Subtract(x=w2526, y=w2527) -> (x-y=w2525:dbl)
                  n1004 = Divide(x=w2525, y=2.0) -> (x/y=w2523:dbl)
                }
                frame "g" {
                  n1005 = Multiply(x=w2531, y=20.0) -> (x*y=w2535:dbl)
                  n1006 = Quotient & Remainder(x=w2535, y=5.0) -> (x-y*floor(x/y)=w2536:dbl)  [unwired: 1 out]
                  n1007 = Subtract(x=w2535, y=w2536) -> (x-y=w2534:dbl)
                  n1008 = Divide(x=w2534, y=20.0) -> (x/y=w2532:dbl)
                }
                frame "daN" {
                  n1009 = Multiply(x=w2540, y=20.0) -> (x*y=w2544:dbl)
                  n1010 = Quotient & Remainder(x=w2544, y=5.0) -> (x-y*floor(x/y)=w2545:dbl)  [unwired: 1 out]
                  n1011 = Subtract(x=w2544, y=w2545) -> (x-y=w2543:dbl)
                  n1012 = Divide(x=w2543, y=20.0) -> (x/y=w2541:dbl)
                }
                frame "cN" {
                }
                frame "KN" {
                  n1013 = Multiply(x=w2552, y=2000.0) -> (x*y=w2555:dbl)
                  n1014 = Quotient & Remainder(x=w2555, y=5.0) -> (x-y*floor(x/y)=w2556:dbl)  [unwired: 1 out]
                  n1015 = Subtract(x=w2555, y=w2556) -> (x-y=w2554:dbl)
                  n1016 = Divide(x=w2554, y=2000.0) -> (x/y=w2551:dbl)
                }
                frame "lb" {
                  n1017 = Multiply(x=w2560, y=10.0) -> (x*y=w2564:dbl)
                  n1018 = Quotient & Remainder(x=w2564, y=5.0) -> (x-y*floor(x/y)=w2565:dbl)  [unwired: 1 out]
                  n1019 = Subtract(x=w2564, y=w2565) -> (x-y=w2563:dbl)
                  n1020 = Divide(x=w2563, y=10.0) -> (x/y=w2561:dbl)
                }
              }
            }
          }
        }
        frame 14 {
          n1021 = case shown="1" w2571 {
            tunnel: [w2577 w2632] -> w2570
            tunnel: [w2576 w2631] -> w2569
            tunnel: w2573 -> [w2575 w2630]
            tunnel: w2572 -> [w2574 w2629]
            frame 0, Default {
              n1022 = case shown="\"lb\"" w2574 {
                tunnel: [w2579 w2587 w2594 w2597 w2604 w2607 w2615] -> w2577
                tunnel: [0 0 0 0 0 2 0] -> w2576
                tunnel: w2575 -> [w2580 w2588 w2594 w2598 w2604 w2608 w2619]
                frame "Kg", Default {
                  n1023 = Absolute Value(x=w2580) -> (abs(x)=w2578:dbl)
                  n1024 = Greater?(x=w2578, y=2.0) -> (0:w2582:bool)
                  n1025 = case shown="False" w2582 {
                    tunnel: w2580 -> [_ w2585]
                    tunnel: [0.0 w2585] -> w2579
                    frame False {
                    }
                    frame True {
                    }
                  }
                }
                frame "N" {
                  n1026 = Absolute Value(x=w2588) -> (abs(x)=w2586:dbl)
                  n1027 = Greater?(x=w2586, y=10.0) -> (0:w2590:bool)
                  n1028 = case shown="False" w2590 {
                    tunnel: w2588 -> [_ w2593]
                    tunnel: [0.0 w2593] -> w2587
                    frame False {
                    }
                    frame True {
                    }
                  }
                }
                frame "g" {
                }
                frame "daN" {
                  n1029 = Absolute Value(x=w2598) -> (abs(x)=w2596:dbl)
                  n1030 = Greater?(x=w2596, y=1.0) -> (0:w2600:bool)
                  n1031 = case shown="False" w2600 {
                    tunnel: w2598 -> [_ w2603]
                    tunnel: [0.0 w2603] -> w2597
                    frame False {
                    }
                    frame True {
                    }
                  }
                }
                frame "cN" {
                }
                frame "KN" {
                  n1032 = Absolute Value(x=w2608) -> (abs(x)=w2606:dbl)
                  n1033 = Greater?(x=w2606, y=0.02) -> (0:w2610:bool)
                  n1034 = case shown="False" w2610 {
                    tunnel: w2608 -> [_ w2613]
                    tunnel: [0.0 w2613] -> w2607
                    frame False {
                    }
                    frame True {
                    }
                  }
                }
                frame "lb" {
                  n1035 = Multiply(x=w2619, y=1.0) -> (x*y=w2622:dbl)
                  n1036 = Quotient & Remainder(x=w2622, y=2.0) -> (x-y*floor(x/y)=w2623:dbl)  [unwired: 1 out]
                  n1037 = Subtract(x=w2622, y=w2623) -> (x-y=w2621:dbl)
                  n1038 = Divide(x=w2621, y=1.0) -> (x/y=w2616:dbl)
                  n1039 = Absolute Value(x=w2616) -> (abs(x)=w2614:dbl)
                  n1040 = Greater?(x=w2614, y=4.0) -> (0:w2618:bool)
                  n1041 = case shown="False" w2618 {
                    tunnel: w2616 -> [_ w2628]
                    tunnel: [0.0 w2628] -> w2615
                    frame False {
                    }
                    frame True {
                    }
                  }
                }
              }
            }
            frame 1 {
              n1042 = case shown="\"KN\"" w2629 {
                tunnel: [w2634 w2642 w2644 w2647 w2655 w2657 w2667] -> w2632
                tunnel: [0 0 0 0 0 2 0] -> w2631
                tunnel: w2630 -> [w2633 w2642 w2644 w2646 w2655 w2658 w2668]
                frame "Kg", Default {
                  n1043 = Multiply(x=w2633, y=1.0) -> (x*y=w2637:dbl)
                  n1044 = Quotient & Remainder(x=w2637, y=5.0) -> (x-y*floor(x/y)=w2638:dbl)  [unwired: 1 out]
                  n1045 = Subtract(x=w2637, y=w2638) -> (x-y=w2636:dbl)
                  n1046 = Divide(x=w2636, y=1.0) -> (x/y=w2634:dbl)
                }
                frame "N" {
                }
                frame "g" {
                }
                frame "daN" {
                  n1047 = Multiply(x=w2646, y=1.0) -> (x*y=w2650:dbl)
                  n1048 = Quotient & Remainder(x=w2650, y=5.0) -> (x-y*floor(x/y)=w2651:dbl)  [unwired: 1 out]
                  n1049 = Subtract(x=w2650, y=w2651) -> (x-y=w2649:dbl)
                  n1050 = Divide(x=w2649, y=1.0) -> (x/y=w2647:dbl)
                }
                frame "cN" {
                }
                frame "KN" {
                  n1051 = Multiply(x=w2658, y=100.0) -> (x*y=w2661:dbl)
                  n1052 = Quotient & Remainder(x=w2661, y=5.0) -> (x-y*floor(x/y)=w2662:dbl)  [unwired: 1 out]
                  n1053 = Subtract(x=w2661, y=w2662) -> (x-y=w2660:dbl)
                  n1054 = Divide(x=w2660, y=100.0) -> (x/y=w2657:dbl)
                }
                frame "lb" {
                  n1055 = Divide(x=w2668, y=10.0) -> (x/y=w2666:dbl)
                  n1056 = Multiply(x=w2666, y=10.0) -> (x*y=w2667:dbl)
                }
              }
            }
          }
        }
        frame 21 {
          n1057 = case shown="0, Default" w2674 {
            tunnel: [w2680 w2735] -> w2673
            tunnel: [w2679 w2734] -> w2672
            tunnel: w2676 -> [w2678 w2733]
            tunnel: w2675 -> [w2677 w2732]
            frame 0, Default {
              n1058 = case shown="\"daN\"" w2677 {
                tunnel: [w2682 w2690 w2697 w2700 w2707 w2710 w2718] -> w2680
                tunnel: [0 0 0 0 0 2 0] -> w2679
                tunnel: w2678 -> [w2683 w2691 w2697 w2701 w2707 w2711 w2722]
                frame "Kg", Default {
                  n1059 = Absolute Value(x=w2683) -> (abs(x)=w2681:dbl)
                  n1060 = Greater?(x=w2681, y=2.0) -> (0:w2685:bool)
                  n1061 = case shown="False" w2685 {
                    tunnel: w2683 -> [_ w2688]
                    tunnel: [0.0 w2688] -> w2682
                    frame False {
                    }
                    frame True {
                    }
                  }
                }
                frame "N" {
                  n1062 = Absolute Value(x=w2691) -> (abs(x)=w2689:dbl)
                  n1063 = Greater?(x=w2689, y=10.0) -> (0:w2693:bool)
                  n1064 = case shown="False" w2693 {
                    tunnel: w2691 -> [_ w2696]
                    tunnel: [0.0 w2696] -> w2690
                    frame False {
                    }
                    frame True {
                    }
                  }
                }
                frame "g" {
                }
                frame "daN" {
                  n1065 = Absolute Value(x=w2701) -> (abs(x)=w2699:dbl)
                  n1066 = Greater?(x=w2699, y=1.0) -> (0:w2703:bool)
                  n1067 = case shown="False" w2703 {
                    tunnel: w2701 -> [_ w2706]
                    tunnel: [0.0 w2706] -> w2700
                    frame False {
                    }
                    frame True {
                    }
                  }
                }
                frame "cN" {
                }
                frame "KN" {
                  n1068 = Absolute Value(x=w2711) -> (abs(x)=w2709:dbl)
                  n1069 = Greater?(x=w2709, y=0.02) -> (0:w2713:bool)
                  n1070 = case shown="False" w2713 {
                    tunnel: w2711 -> [_ w2716]
                    tunnel: [0.0 w2716] -> w2710
                    frame False {
                    }
                    frame True {
                    }
                  }
                }
                frame "lb" {
                  n1071 = Multiply(x=w2722, y=1.0) -> (x*y=w2725:dbl)
                  n1072 = Quotient & Remainder(x=w2725, y=2.0) -> (x-y*floor(x/y)=w2726:dbl)  [unwired: 1 out]
                  n1073 = Subtract(x=w2725, y=w2726) -> (x-y=w2724:dbl)
                  n1074 = Divide(x=w2724, y=1.0) -> (x/y=w2719:dbl)
                  n1075 = Absolute Value(x=w2719) -> (abs(x)=w2717:dbl)
                  n1076 = Greater?(x=w2717, y=4.0) -> (0:w2721:bool)
                  n1077 = case shown="False" w2721 {
                    tunnel: w2719 -> [_ w2731]
                    tunnel: [0.0 w2731] -> w2718
                    frame False {
                    }
                    frame True {
                    }
                  }
                }
              }
            }
            frame 1 {
              n1078 = case shown="\"KN\"" w2732 {
                tunnel: [w2737 w2745 w2752 w2755 w2762 w2765 w2773] -> w2735
                tunnel: [0 0 0 0 0 2 0] -> w2734
                tunnel: w2733 -> [w2738 w2746 w2752 w2756 w2762 w2766 w2777]
                frame "Kg", Default {
                  n1079 = Absolute Value(x=w2738) -> (abs(x)=w2736:dbl)
                  n1080 = Greater?(x=w2736, y=2.0) -> (0:w2740:bool)
                  n1081 = case shown="False" w2740 {
                    tunnel: w2738 -> [_ w2743]
                    tunnel: [0.0 w2743] -> w2737
                    frame False {
                    }
                    frame True {
                    }
                  }
                }
                frame "N" {
                  n1082 = Absolute Value(x=w2746) -> (abs(x)=w2744:dbl)
                  n1083 = Greater?(x=w2744, y=10.0) -> (0:w2748:bool)
                  n1084 = case shown="False" w2748 {
                    tunnel: w2746 -> [_ w2751]
                    tunnel: [0.0 w2751] -> w2745
                    frame False {
                    }
                    frame True {
                    }
                  }
                }
                frame "g" {
                }
                frame "daN" {
                  n1085 = Absolute Value(x=w2756) -> (abs(x)=w2754:dbl)
                  n1086 = Greater?(x=w2754, y=1.0) -> (0:w2758:bool)
                  n1087 = case shown="False" w2758 {
                    tunnel: w2756 -> [_ w2761]
                    tunnel: [0.0 w2761] -> w2755
                    frame False {
                    }
                    frame True {
                    }
                  }
                }
                frame "cN" {
                }
                frame "KN" {
                  n1088 = Absolute Value(x=w2766) -> (abs(x)=w2764:dbl)
                  n1089 = Greater?(x=w2764, y=0.02) -> (0:w2768:bool)
                  n1090 = case shown="False" w2768 {
                    tunnel: w2766 -> [_ w2771]
                    tunnel: [0.0 w2771] -> w2765
                    frame False {
                    }
                    frame True {
                    }
                  }
                }
                frame "lb" {
                  n1091 = Multiply(x=w2777, y=1.0) -> (x*y=w2780:dbl)
                  n1092 = Quotient & Remainder(x=w2780, y=2.0) -> (x-y*floor(x/y)=w2781:dbl)  [unwired: 1 out]
                  n1093 = Subtract(x=w2780, y=w2781) -> (x-y=w2779:dbl)
                  n1094 = Divide(x=w2779, y=1.0) -> (x/y=w2774:dbl)
                  n1095 = Absolute Value(x=w2774) -> (abs(x)=w2772:dbl)
                  n1096 = Greater?(x=w2772, y=4.0) -> (0:w2776:bool)
                  n1097 = case shown="False" w2776 {
                    tunnel: w2774 -> [_ w2786]
                    tunnel: [0.0 w2786] -> w2773
                    frame False {
                    }
                    frame True {
                    }
                  }
                }
              }
            }
          }
        }
        frame 15 {
          n1098 = case shown="1" w2789 {
            tunnel: [w2795 w2865] -> w2787
            tunnel: [w2794 w2864] -> w2788
            tunnel: w2791 -> [w2793 w2863]
            tunnel: w2790 -> [w2792 w2862]
            frame 0, Default {
              n1099 = case shown="\"lb\"" w2792 {
                tunnel: [w2797 w2811 w2813 w2816 w2830 w2833 w2848] -> w2795
                tunnel: [0 0 0 0 0 2 1] -> w2794
                tunnel: w2793 -> [w2801 w2811 w2813 w2820 w2830 w2837 w2852]
                frame "Kg", Default {
                  n1100 = Multiply(x=w2801, y=1.0) -> (x*y=w2804:dbl)
                  n1101 = Quotient & Remainder(x=w2804, y=2.0) -> (x-y*floor(x/y)=w2805:dbl)  [unwired: 1 out]
                  n1102 = Subtract(x=w2804, y=w2805) -> (x-y=w2803:dbl)
                  n1103 = Divide(x=w2803, y=1.0) -> (x/y=w2798:dbl)
                  n1104 = Absolute Value(x=w2798) -> (abs(x)=w2796:dbl)
                  n1105 = Greater?(x=w2796, y=4.0) -> (0:w2800:bool)
                  n1106 = case shown="False" w2800 {
                    tunnel: w2798 -> [_ w2810]
                    tunnel: [0.0 w2810] -> w2797
                    frame False {
                    }
                    frame True {
                    }
                  }
                }
                frame "N" {
                }
                frame "g" {
                }
                frame "daN" {
                  n1107 = Multiply(x=w2820, y=1.0) -> (x*y=w2823:dbl)
                  n1108 = Quotient & Remainder(x=w2823, y=2.0) -> (x-y*floor(x/y)=w2824:dbl)  [unwired: 1 out]
                  n1109 = Subtract(x=w2823, y=w2824) -> (x-y=w2822:dbl)
                  n1110 = Divide(x=w2822, y=1.0) -> (x/y=w2817:dbl)
                  n1111 = Absolute Value(x=w2817) -> (abs(x)=w2815:dbl)
                  n1112 = Greater?(x=w2815, y=4.0) -> (0:w2819:bool)
                  n1113 = case shown="False" w2819 {
                    tunnel: w2817 -> [_ w2829]
                    tunnel: [0.0 w2829] -> w2816
                    frame False {
                    }
                    frame True {
                    }
                  }
                }
                frame "cN" {
                }
                frame "KN" {
                  n1114 = Multiply(x=w2837, y=100.0) -> (x*y=w2840:dbl)
                  n1115 = Quotient & Remainder(x=w2840, y=2.0) -> (x-y*floor(x/y)=w2841:dbl)  [unwired: 1 out]
                  n1116 = Subtract(x=w2840, y=w2841) -> (x-y=w2839:dbl)
                  n1117 = Divide(x=w2839, y=100.0) -> (x/y=w2834:dbl)
                  n1118 = Absolute Value(x=w2834) -> (abs(x)=w2832:dbl)
                  n1119 = Greater?(x=w2832, y=0.04) -> (0:w2836:bool)
                  n1120 = case shown="False" w2836 {
                    tunnel: w2834 -> [_ w2846]
                    tunnel: [0.0 w2846] -> w2833
                    frame False {
                    }
                    frame True {
                    }
                  }
                }
                frame "lb" {
                  n1121 = Multiply(x=w2852, y=1.0) -> (x*y=w2855:dbl)
                  n1122 = Quotient & Remainder(x=w2855, y=5.0) -> (x-y*floor(x/y)=w2856:dbl)  [unwired: 1 out]
                  n1123 = Subtract(x=w2855, y=w2856) -> (x-y=w2854:dbl)
                  n1124 = Divide(x=w2854, y=1.0) -> (x/y=w2849:dbl)
                  n1125 = Absolute Value(x=w2849) -> (abs(x)=w2847:dbl)
                  n1126 = Greater?(x=w2847, y=10.0) -> (0:w2851:bool)
                  n1127 = case shown="False" w2851 {
                    tunnel: w2849 -> [_ w2861]
                    tunnel: [0.0 w2861] -> w2848
                    frame False {
                    }
                    frame True {
                    }
                  }
                }
              }
            }
            frame 1 {
              n1128 = case shown="\"lb\"" w2862 {
                tunnel: [w2866 w2872 w2874 w2876 w2882 w2884 w2887] -> w2865
                tunnel: [0 0 0 0 0 1 0] -> w2864
                tunnel: w2863 -> [w2867 w2872 w2874 w2877 w2882 w2884 w2886]
                frame "Kg", Default {
                  w2868 = 10.0 ("y")
                  n1129 = Divide(x=w2867, y=w2868) -> (x/y=w2869:dbl)
                  n1130 = To Word Integer(number=w2869) -> (16bit integer=w2870:i16)
                  n1131 = Multiply(x=w2870, y=w2868) -> (x*y=w2866:dbl)
                }
                frame "N" {
                }
                frame "g" {
                }
                frame "daN" {
                  w2880 = 10.0 ("y")
                  n1132 = Divide(x=w2877, y=w2880) -> (x/y=w2879:dbl)
                  n1133 = To Word Integer(number=w2879) -> (16bit integer=w2878:i16)
                  n1134 = Multiply(x=w2878, y=w2880) -> (x*y=w2876:dbl)
                }
                frame "cN" {
                }
                frame "KN" {
                }
                frame "lb" {
                  n1135 = Divide(x=w2886, y=20.0) -> (x/y=w2890:dbl)
                  n1136 = Quotient & Remainder(x=w2890, y=5.0) -> (x-y*floor(x/y)=w2891:dbl)  [unwired: 1 out]
                  n1137 = Subtract(x=w2890, y=w2891) -> (x-y=w2889:dbl)
                  n1138 = Multiply(x=w2889, y=20.0) -> (x*y=w2887:dbl)
                }
              }
            }
          }
        }
        frame 16, 23 {
          n1139 = case shown="1" w2897 {
            tunnel: [w2903 w2970] -> w2896
            tunnel: [w2902 w2969] -> w2895
            tunnel: w2899 -> [w2901 w2968]
            tunnel: w2898 -> [w2900 w2967]
            frame 0, Default {
              n1140 = case shown="\"g\"" w2900 {
                tunnel: [w2905 w2919 w2921 w2924 w2938 w2941 w2961] -> w2903
                tunnel: [0 0 0 1 0 2 0] -> w2902
                tunnel: w2901 -> [w2909 w2919 w2921 w2928 w2938 w2945 w2956]
                frame "Kg", Default {
                  n1141 = Multiply(x=w2909, y=1.0) -> (x*y=w2912:dbl)
                  n1142 = Quotient & Remainder(x=w2912, y=5.0) -> (x-y*floor(x/y)=w2913:dbl)  [unwired: 1 out]
                  n1143 = Subtract(x=w2912, y=w2913) -> (x-y=w2911:dbl)
                  n1144 = Divide(x=w2911, y=1.0) -> (x/y=w2906:dbl)
                  n1145 = Absolute Value(x=w2906) -> (abs(x)=w2904:dbl)
                  n1146 = Greater?(x=w2904, y=10.0) -> (0:w2908:bool)
                  n1147 = case shown="False" w2908 {
                    tunnel: w2906 -> [_ w2918]
                    tunnel: [0.0 w2918] -> w2905
                    frame False {
                    }
                    frame True {
                    }
                  }
                }
                frame "N" {
                }
                frame "g" {
                }
                frame "daN" {
                  n1148 = Multiply(x=w2928, y=1.0) -> (x*y=w2931:dbl)
                  n1149 = Quotient & Remainder(x=w2931, y=5.0) -> (x-y*floor(x/y)=w2932:dbl)  [unwired: 1 out]
                  n1150 = Subtract(x=w2931, y=w2932) -> (x-y=w2930:dbl)
                  n1151 = Divide(x=w2930, y=1.0) -> (x/y=w2925:dbl)
                  n1152 = Absolute Value(x=w2925) -> (abs(x)=w2923:dbl)
                  n1153 = Greater?(x=w2923, y=10.0) -> (0:w2927:bool)
                  n1154 = case shown="False" w2927 {
                    tunnel: w2925 -> [_ w2937]
                    tunnel: [0.0 w2937] -> w2924
                    frame False {
                    }
                    frame True {
                    }
                  }
                }
                frame "cN" {
                }
                frame "KN" {
                  n1155 = Multiply(x=w2945, y=100.0) -> (x*y=w2948:dbl)
                  n1156 = Quotient & Remainder(x=w2948, y=5.0) -> (x-y*floor(x/y)=w2949:dbl)  [unwired: 1 out]
                  n1157 = Subtract(x=w2948, y=w2949) -> (x-y=w2947:dbl)
                  n1158 = Divide(x=w2947, y=100.0) -> (x/y=w2942:dbl)
                  n1159 = Absolute Value(x=w2942) -> (abs(x)=w2940:dbl)
                  n1160 = Greater?(x=w2940, y=0.1) -> (0:w2944:bool)
                  n1161 = case shown="False" w2944 {
                    tunnel: w2942 -> [_ w2954]
                    tunnel: [0.0 w2954] -> w2941
                    frame False {
                    }
                    frame True {
                    }
                  }
                }
                frame "lb" {
                  w2959 = 10.0 ("y")
                  n1162 = Divide(x=w2956, y=w2959) -> (x/y=w2958:dbl)
                  n1163 = To Word Integer(number=w2958) -> (16bit integer=w2957:i16)
                  n1164 = Multiply(x=w2957, y=w2959) -> (x*y=w2955:dbl)
                  n1165 = Absolute Value(x=w2955) -> (abs(x)=w2960:dbl)
                  n1166 = Greater?(x=w2960, y=20.0) -> (0:w2963:bool)
                  n1167 = case shown="False" w2963 {
                    tunnel: w2955 -> [_ w2966]
                    tunnel: [0.0 w2966] -> w2961
                    frame False {
                    }
                    frame True {
                    }
                  }
                }
              }
            }
            frame 1 {
              n1168 = case shown="\"daN\"" w2967 {
                tunnel: [w2972 w2980 w2982 w2984 w2993 w2995 w3005] -> w2970
                tunnel: [0 1 0 0 0 1 0] -> w2969
                tunnel: w2968 -> [w2971 w2980 w2982 w2985 w2993 w2996 w3004]
                frame "Kg", Default {
                  n1169 = Divide(x=w2971, y=10.0) -> (x/y=w2975:dbl)
                  n1170 = Quotient & Remainder(x=w2975, y=2.0) -> (x-y*floor(x/y)=w2976:dbl)  [unwired: 1 out]
                  n1171 = Subtract(x=w2975, y=w2976) -> (x-y=w2974:dbl)
                  n1172 = Multiply(x=w2974, y=10.0) -> (x*y=w2972:dbl)
                }
                frame "N" {
                }
                frame "g" {
                }
                frame "daN" {
                  n1173 = Divide(x=w2985, y=10.0) -> (x/y=w2988:dbl)
                  n1174 = Quotient & Remainder(x=w2988, y=2.0) -> (x-y*floor(x/y)=w2989:dbl)  [unwired: 1 out]
                  n1175 = Subtract(x=w2988, y=w2989) -> (x-y=w2987:dbl)
                  n1176 = Multiply(x=w2987, y=10.0) -> (x*y=w2984:dbl)
                }
                frame "cN" {
                }
                frame "KN" {
                  n1177 = Multiply(x=w2996, y=10.0) -> (x*y=w2999:dbl)
                  n1178 = Quotient & Remainder(x=w2999, y=2.0) -> (x-y*floor(x/y)=w3000:dbl)  [unwired: 1 out]
                  n1179 = Subtract(x=w2999, y=w3000) -> (x-y=w2998:dbl)
                  n1180 = Divide(x=w2998, y=10.0) -> (x/y=w2995:dbl)
                }
                frame "lb" {
                  n1181 = Divide(x=w3004, y=10.0) -> (x/y=w3008:dbl)
                  n1182 = Quotient & Remainder(x=w3008, y=5.0) -> (x-y*floor(x/y)=w3009:dbl)  [unwired: 1 out]
                  n1183 = Subtract(x=w3008, y=w3009) -> (x-y=w3007:dbl)
                  n1184 = Multiply(x=w3007, y=10.0) -> (x*y=w3005:dbl)
                }
              }
            }
          }
        }
      }
    }
    frame #1 {
      n1185 = property on="ValorOut" class="DigNum (strict)"("Value"=w3014) -> ()  [unwired: 2 in, 2 out]
      "NDecimals" <- w3013
    }
  }
